vi "MultiQ_09_DataSwitch.vi"() -> ()   [LabVIEW 2021]
doc: "I. Description:\nThis example demonstrates how to acquire a finite amount of data (waveform) using the DAQ device's internal clock.\n\nII. Instructions for Running:\n1. Select the physical channel to correspond to where your signal is input on the DAQ device.\n2. Enter the minimum and maximum voltages.\nNote: For better accuracy try to match the input range to the expected voltage level of the measured signal.\n3. Select the number of samples to acquire.\n4. Set the rate of the acquisition\nNote: The rate should be AT LEAST twice as fast as the maximum frequency component of the signal being acquired.\n\nIII. Block Diagram Steps:\n Steps: \n1. Create an empty task.\n2. Create an analog input voltage channel. Use the DAQmx Base configuration Utility (Tools Menu) to determine the DAQ device name. \n3. Set the rate for the sample clock. Additionally, define the sample mode to be finite and set the number of samples to be acquired per channel.\n4. Call the Start VI to start the acquisition.\n5. Use the Read VI to measure multiple samples from N Channels on the device. Set a timeout so an error is returned if the samples are not returned in the specified time limit\n6. Stop the Analog Input Task.\n7. Call the Clear Task VI to clear the Task.\n8. Use the popup dialog box to display an error if any.\n \nIV. I/O Connections Overview:\nMake sure your signal input terminal matches the Physical Channel I/O Control. For further connection information, refer to your hardware reference manual."
uses:
  <vilib>/Utility/error.llb/DialogType.ctl
  <vilib>/DAQmx/write.llb/DAQmx Write (Analog 2D DBL NChan NSamp).vi
  <vilib>/measure/maspectr.llb/FFT Power Spectrum and PSD for 1 Chan.vi
  <vilib>/DAQmx/configure/timing.llb/DAQmx Timing (Sample Clock).vi
  <vilib>/DAQmx/miscellaneous.llb/DAQmx Fill In Error Info.vi
  <vilib>/Analysis/2dsp.llb/Decimate (continuous, DBL).vi
  <vilib>/DAQmx/create/channels.llb/DAQmx Create Channel (AI-Voltage-Basic).vi
  <vilib>/measure/macond.llb/IIR Filter for 1 Chan.vi
  <vilib>/DAQmx/configure/trigger.llb/DAQmx Start Trigger (Digital Edge).vi
  <vilib>/DAQmx/create/channels.llb/DAQmx Create Channel (AO-Voltage-Basic).vi
  <vilib>/DAQmx/read.llb/DAQmx Read (Analog 2D DBL NChan NSamp).vi
  <vilib>/measure/NI_MAPro.lvlib
  <vilib>/measure/NI_MABase.lvlib
  <vilib>/Analysis/NI_AALPro.lvlib
  <resource>/objmgr/daqmx.rc
panel:
  out "Nodal Modes":dbl[](array[numeric])=[1092.3, 1649.9, 2505.8]
  out "PlotLabelSize":i32[](array[numeric])
  out "PlotModeSize":i32[](array[numeric])
  out "PlotFreqArray":dbl[][](array[numeric])
  out "PlotLabelArray":string[][](array[string])
  out "Shear Modes":dbl[](array[numeric])=[1092.3, 1649.9, 2505.8]
  out "All Modes":dbl[](array[numeric])=[1092.3, 1649.9, 2505.8]
  out "Modes 10-12":dbl[](array[numeric])=[10072.0, 11259.0, 12454.0]
  out "Modes 7-9":dbl[](array[numeric])=[6683.3, 7225.3, 9346.1]
  in  "Sample Modes":u16(ring)=1 items=["All Modes", "Shear Modes"]
  out "Plot7Label":string="Mode 15: 15961 Hz"
  out "Plot5Label":string="Mode 9: 9346 Hz"
  out "Plot3Label":string="Mode 5: 4361 Hz"
  out "Plot1Label":string="Mode 1: 1092 Hz"
  out "Plot8Label":string="Mode 18: 19859 Hz"
  out "Plot6Label":string="Mode 12: 12454 Hz"
  out "Plot4Label":string="Mode 6: 6645 Hz"
  out "Plot2Label":string="Mode 3: 2506 Hz"
  in  "Ring":u16(ring) items=["EXCITE", "ACQUIRE", "X-Y"]
  in  "Max Value":dbl=10.0 format="%#_13g"
  in  "Min Value":dbl=-10.0 format="%#_13g"
  out "Modes 4-6":dbl[](array[numeric])=[3847.7, 4361.2, 6645.1]
  out "Modes 1-3":dbl[](array[numeric])=[1092.3, 1649.9, 2505.8]
  out "Converted Data Size":i32[](array[numeric])
  out "Raw Data Size":i32[](array[numeric])
  in  "Input Data Type":u16(ring) items=["X Y SUM", "Q 1+/- -- 4+/-", "Q 1-4"]
  in  "Mode Scale":dbl=1.0 min=0.5 max=2.0
  in  "Range (%)":dbl=1.0
  in  "Pressure (t)":sgl=1e-06
  in  "LeverArm (m)":dbl=1.0 min=1.0 max=10000.0
  in  "ADC Range":u16(ring)=6 items=["±0.1 V", "±0.2 V", "±0.5 V", "±1 V", "±2 V", "±5 V", "±10 V"]
  out "PlotLimit":u64
  out "Plot":i32
  in  "Type":u16(ring)=1 items=["Power Spectrum", "PS Density"]
  in  "Unit":u16(ring)=3 items=["Volts", "mRad (full)", "mRad (o2)", "mRad (o1)"]
  in  "Averaging":T1={"Averaging"=enum."No averaging", "weighting mode"=enum."Linear", "number of averages"=10} {"number of averages" min=1 step=1}
  out "Progress":u8(slide) scale=0.0..100.0
  in  "Who":string(combo)="SP"
  in  "fMinPlot":dbl=0.5
  in  "fMaxPlot":dbl=15.0 min=1.0 max=100.0
  in  "Substrate":u16(ring)=1 items=["Silica: 75 x 0.3 mm", "Silica: 75 x 1.0 mm", "Silica: 75 x 2.54 mm"]
  in  "Oversample":bool=TRUE
  in  "fOversample":dbl=50.0 format="%#_13g"
  in  "Span":u32(ring)=60 items=["20 s"=20, "40 s"=40, "1 min"=60, "3 min"=180, "5 min"=300]
  in  "Offset (V)":sgl=2.0
  in  "Ampl. (V)":sgl=2.0
  out "NAve":dbl format="%#_13g"
  out "ADCScale":dbl format="%#_13g"
  out "SizeTimeSeries":i32
  out "BufferPeriod":dbl format="%#_13g"
  out "PSD X":cluster{"f0":dbl, "df":dbl, dbl[][]}(graph)
  out "PlotUnitIndex":u16
  out "DataFilePath":path
  out "fSampleAcquire":dbl format="%#_13g"
  out "NDataPointsOutput":u64
  out "DeltaTOutput":dbl format="%#_13g"
  out "fSampleOutput":dbl format="%#_13g"
  out "DecimFactor":u32
  in  "Comment":string
  out "WriteNumber":i32
  out "WriteLimit":i32
  out "Step":i32
  out "Location":string
  out "PathAtOpen":path
  out "PathAtClose":path
  out "RunLight":bool
  in  "Temp Path":path
  in  "stop":bool
  out "Plot8":cluster{"f0":dbl, "df":dbl, dbl[][]}(graph)
  out "Plot7":cluster{"f0":dbl, "df":dbl, dbl[][]}(graph)
  out "WriteNewHeader":bool
  out "TempFilePath":path
  out "RunPeriod":dbl format="%#_13g"
  out "NDataPointsAcquire":u64
  out "nPlotPerRun":u64
  out "InitialArray":dbl[][](array[numeric])
  out "time vector":dbl[](array[numeric])
  out "ReZero":dbl[][](array[numeric])
  out "df":dbl format="%#_13g"
  out "PlotPeriod":dbl format="%#_13g"
  in  "Run Duration (s)":u32=100 caption="Duration (s)"
  in  "Run Number":i8=1
  in  "∆f (Hz)":u32(ring)=1 items=["1.00"=1, "0.50"=2, "0.25"=4, "0.10"=10]
  in  "Excite":bool
  out "# Elements Response Queue":i32
  out "BufferPeriod ms":u32
  out "# Elements Drive Queue":i32
  out "High Pass IIR filter specs":T2={"Topology"=enum."Butterworth", "Type"=enum."Bandpass", "Order"=7, "Lower Fc"=2000.0, "Upper Fc"=3800.0, "PB Ripple"=0.025, "SB Attenuation"=90.0}
  out "DeltaTAcquire":dbl format="%#_13g"
  out "BufferPoints":u32
  out "PlotPoints":u32
  out "nBufferPerPlot":u32
  out "fMaxPlotHz":dbl format="%#_13g"
  out "fMinPlotHz":dbl format="%#_13g"
  out "Plot6":cluster{"f0":dbl, "df":dbl, dbl[][]}(graph)
  out "Plot5":cluster{"f0":dbl, "df":dbl, dbl[][]}(graph)
  out "Plot4":cluster{"f0":dbl, "df":dbl, dbl[][]}(graph)
  out "Plot3":cluster{"f0":dbl, "df":dbl, dbl[][]}(graph)
  out "Plot2":cluster{"f0":dbl, "df":dbl, dbl[][]}(graph)
  out "Plot1":cluster{"f0":dbl, "df":dbl, dbl[][]}(graph)
  in  "Start":bool
  out "PSD Y":cluster{"f0":dbl, "df":dbl, dbl[][]}(graph) caption="Measurement"
  out "File":string
  in  "Path":path caption="File Name"
  in  "Label":string
  in  "Name":string
  out "HTML \nTitle":string
  out "Start Time":timestamp
  out "Write Light":bool
  in  "AutoSave":bool=TRUE
  in  "Manual Save":bool=TRUE caption="Saving Data"
  out "Out":path caption="File Name Out"
  in  "QUIT":bool
  # "Acquire"
  # "Multi Q\nVer 0.9.5.0 • July 2021\nSteve Penn"
  # "Sample"
  # "Comment"
  # "Frequency"
  # "kHz"
  # ":"
  # "Oversample"
  # "kHz"
  # "PLOT:"
  # "Mode Plots:"
  # "PSD Y / Excitation"
  # "/"
  # "Averaging"
  # "Drive"
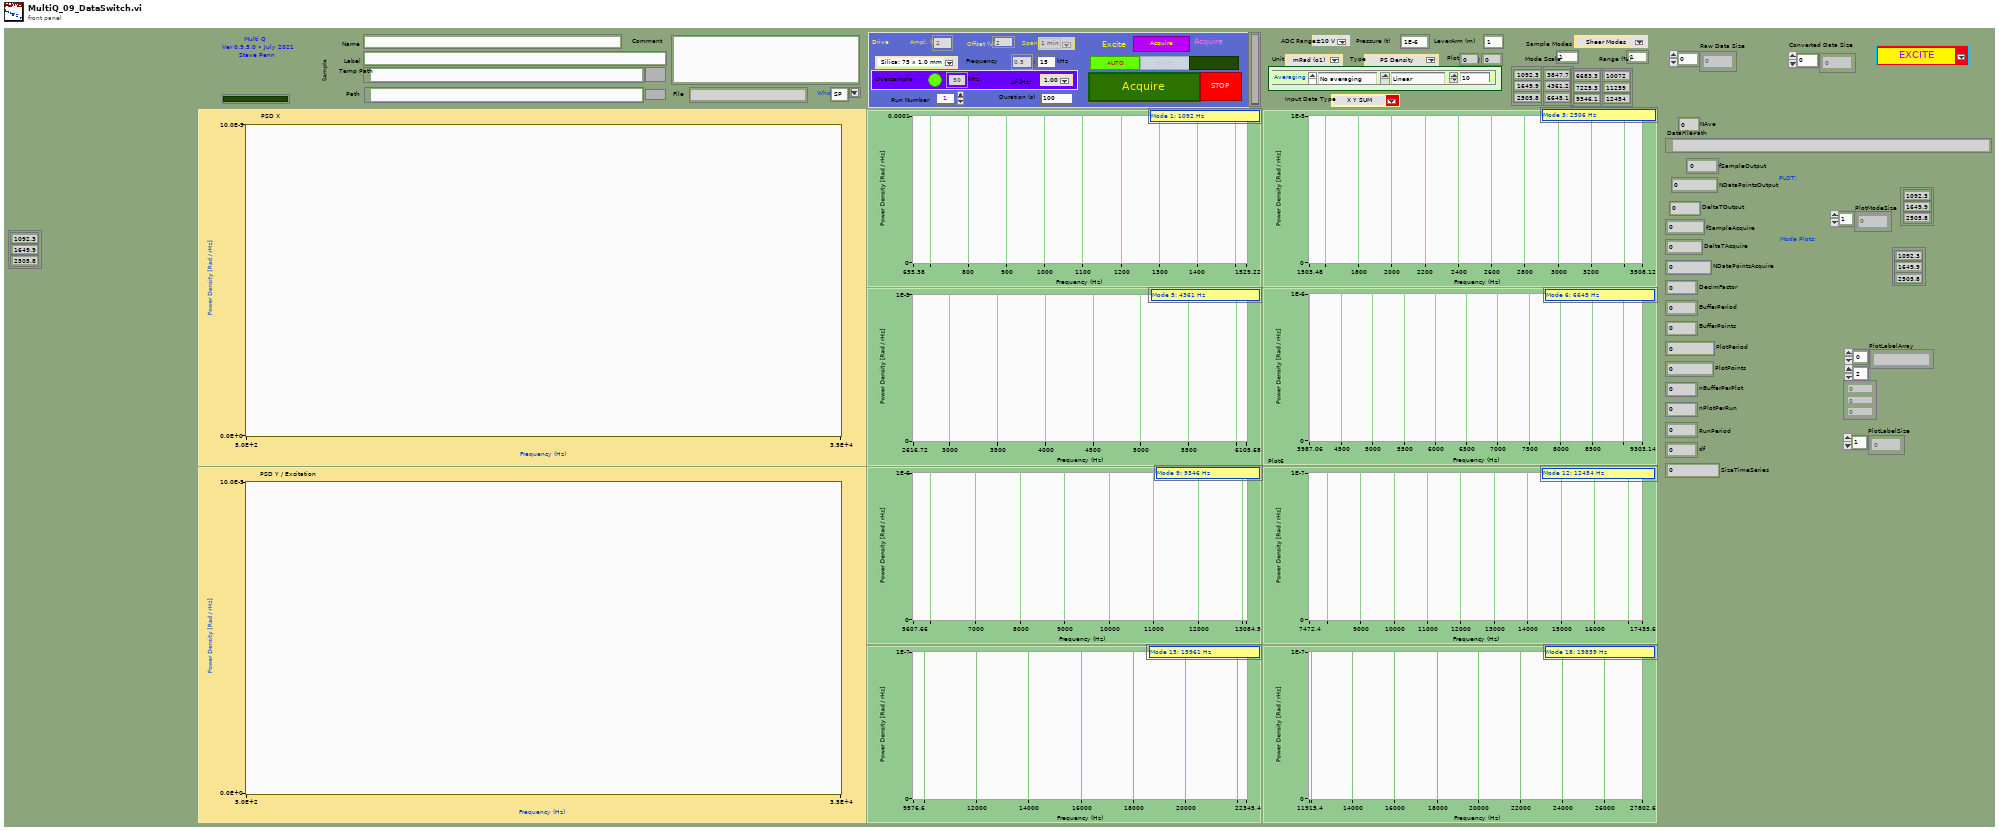
[diagram p1: front panel]
types:
  T1 = cluster{"Averaging":enum16{"No averaging", "Vector averaging", "RMS averaging", "Peak hold"}, "weighting mode":enum16{"Linear", "Exponential"}, "number of averages":u32}
  T2 = cluster{"Topology":enum16{"Off", "Butterworth", "Chebyshev", "Inverse Chebyshev", "Elliptic", "Bessel"}, "Type":enum16{"Lowpass", "Highpass", "Bandpass", "Bandstop"}, "Order":i32, "Lower Fc":dbl, "Upper Fc":dbl, "PB Ripple":dbl, "SB Attenuation":dbl}
  T3 = enum16{"Off", "Butterworth", "Chebyshev", "Inverse Chebyshev", "Elliptic", "Bessel"}
  T4 = enum16{"Lowpass", "Highpass", "Bandpass", "Bandstop"}
  T5 = enum8{"open", "replace", "create", "open or create", "replace or create", "replace or create with confirmation"}
  T6 = enum16{"No averaging", "Vector averaging", "RMS averaging", "Peak hold"}
  T7 = cluster{"Averaging":enum16{"No averaging", "Vector averaging", "RMS averaging", "Peak hold"}, "weighting mode":enum16{"Linear", "Exponential"}, "weighting mode":u64}
  T8 = typedef "DialogType.ctl" = u16
  T9 = enum16{"Left Button", "Center Button", "Right Button", "Window Close"}
  T10 = cluster{"Averaging":enum16{"No averaging", "Vector averaging", "RMS averaging", "Peak hold"}, "weighting mode":enum16{"Linear", "Exponential"}, "Value":u64}
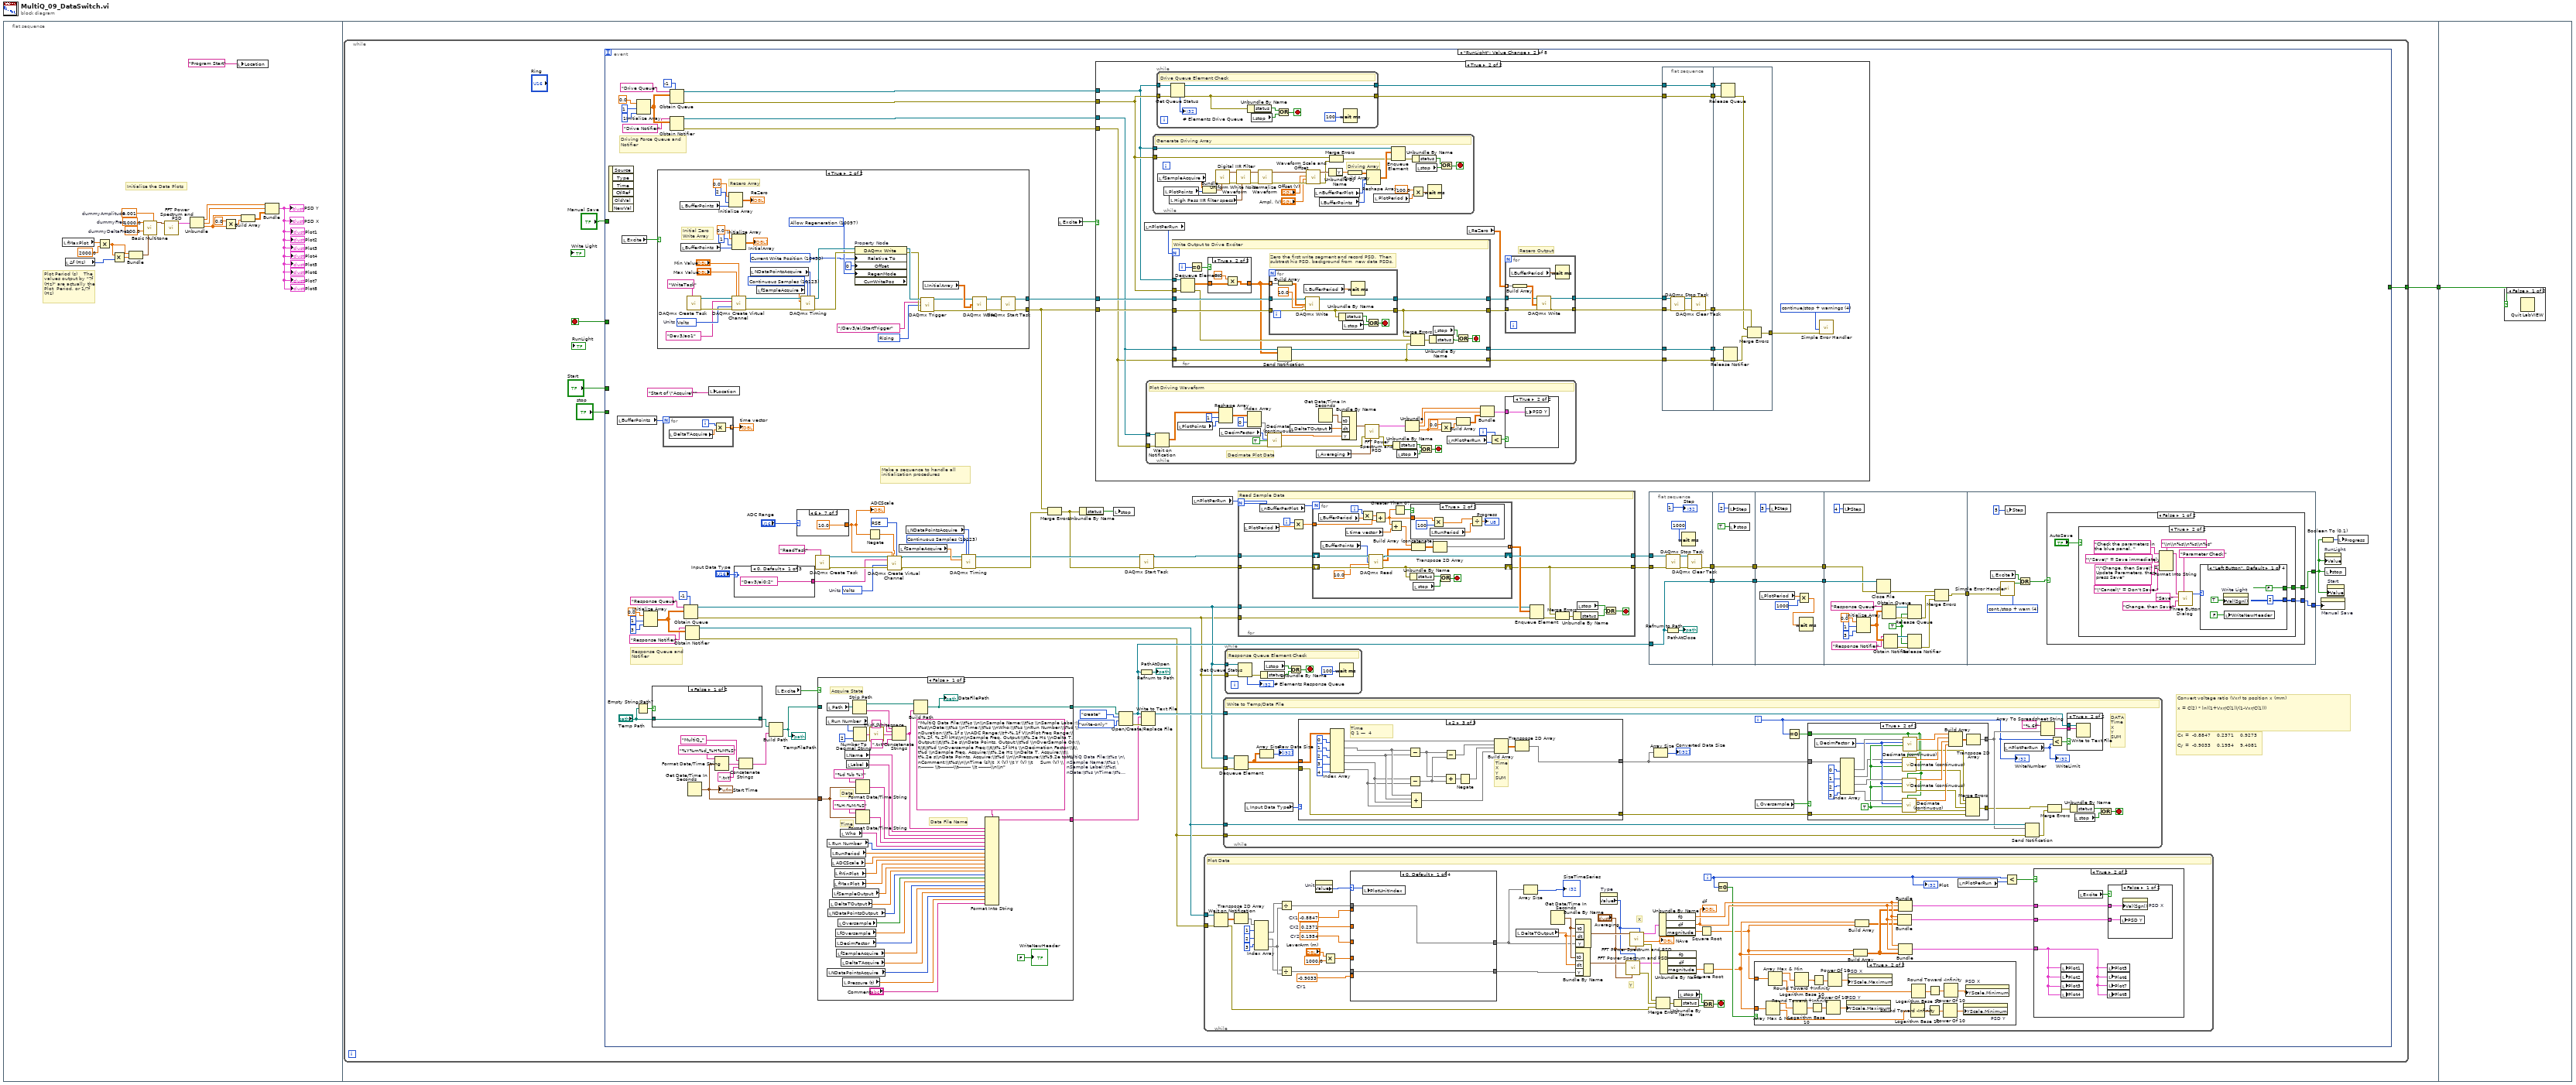
[diagram p0: block diagram]
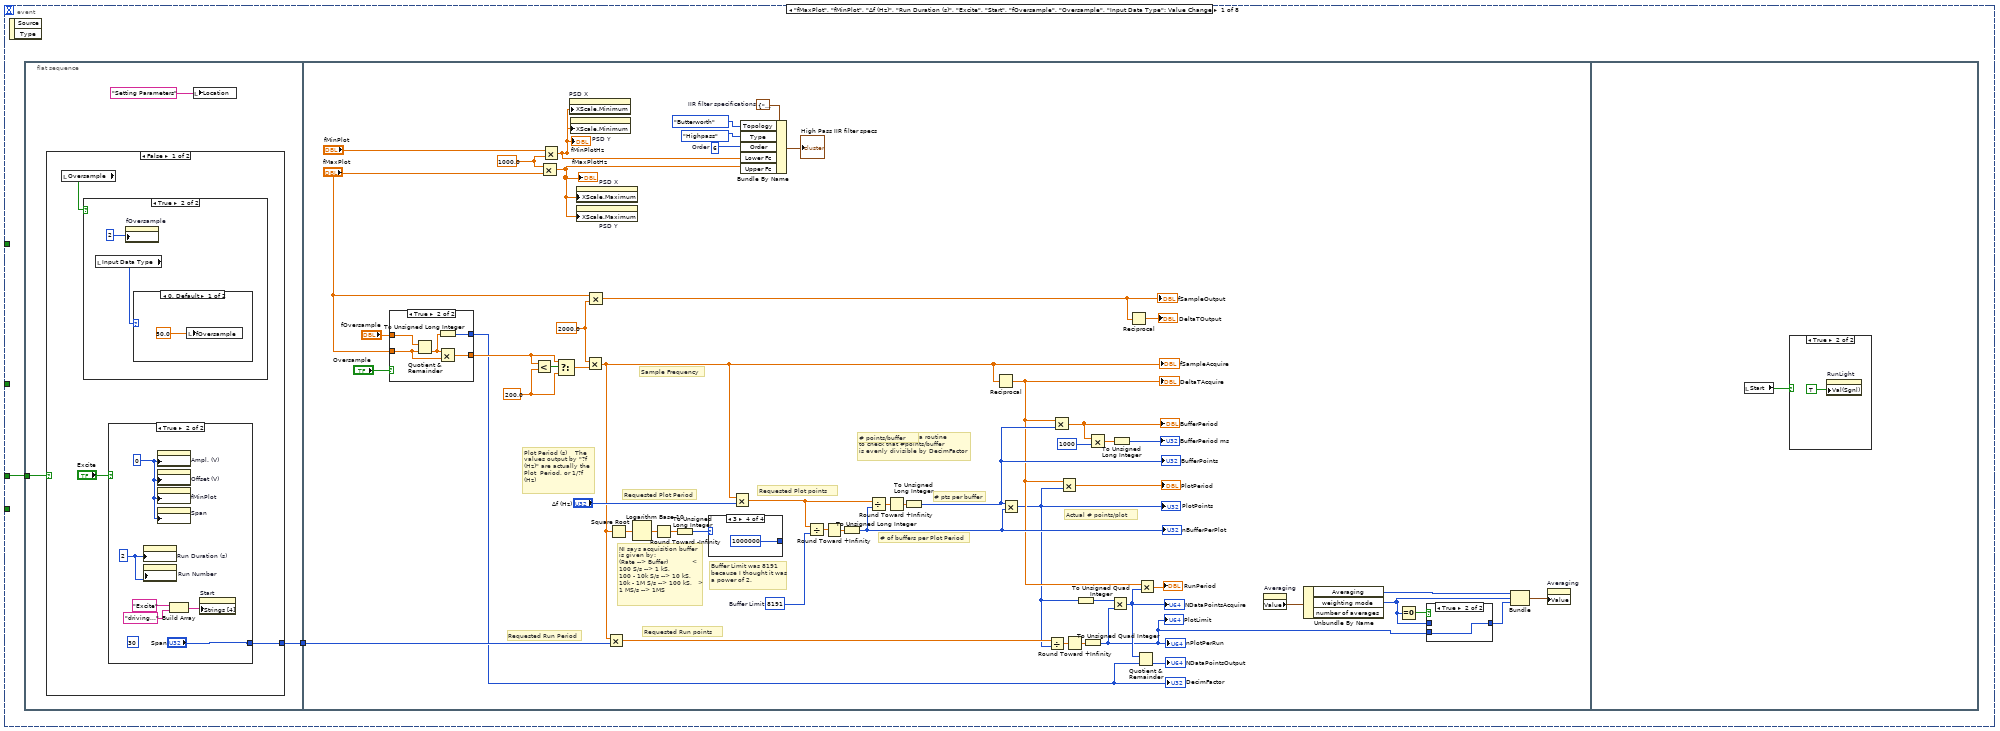
[diagram p2: hidden frame]
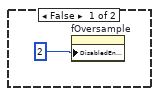
[diagram p3: hidden frame]
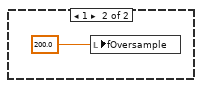
[diagram p4: hidden frame]
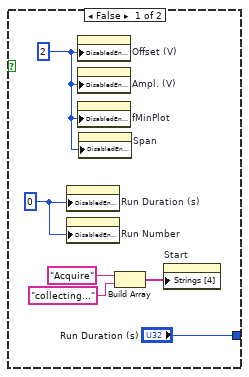
[diagram p5: hidden frame]
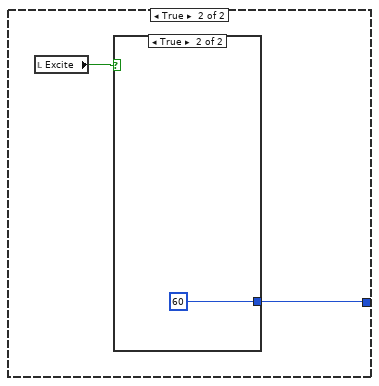
[diagram p6: hidden frame]
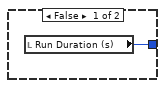
[diagram p7: hidden frame]
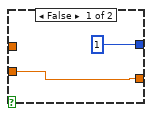
[diagram p9: hidden frame]
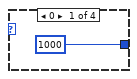
[diagram p10: hidden frame]
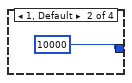
[diagram p11: hidden frame]
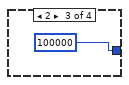
[diagram p12: hidden frame]
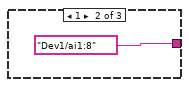
[diagram p14: hidden frame]
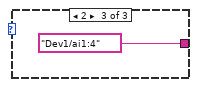
[diagram p15: hidden frame]
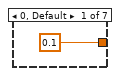
[diagram p16: hidden frame]
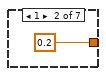
[diagram p17: hidden frame]
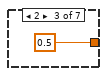
[diagram p18: hidden frame]
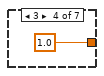
[diagram p19: hidden frame]
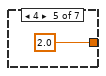
[diagram p20: hidden frame]
diagram:
  n1 = flat-sequence {
    tunnel: [w21] -> w1
    tunnel: w1 -> [w1121]
    frame #0 {
      w4 = 0.001  # dummyAmplitude
      w2 = 100.0  # dummyDeltaFreq
      w3 = 1000.0  # dummyFreq
      # "Initialize the Data Plots"
      # "Plot Period (s)    The values output by \"?f (Hz)\" are actually the Plot  Period, or 1/?f (Hz)"
      n2 = local read "fMaxPlot"() -> (w9:dbl)
      n3 = local read "∆f (Hz)"() -> (w8:u32)
      n4 = Multiply(x=w9, y=2000.0) -> (x*y=w6:dbl)
      n5 = Multiply(x=w6, y=w8) -> (x*y=w7:dbl)
      n6 = Bundle(w6, w7) -> (w19:cluster{dbl, dbl})  [unwired: 1 in]
      n7 = call <vilib>:"Basic Multitone.vi"("start frequency"=w3, "amplitude"=w4, "delta frequency"=w2, "sampling info"=w19) -> ("signal out"=w18:waveform(dbl))  [unwired: 8 in, 3 out]
      n8 = call-poly <vilib>:"FFT Power Spectrum and PSD.vi"("time signal"=w18) -> ("Power Spectrum / PSD"=w11:cluster{"f0":dbl, "df":dbl, "magnitude":dbl[]})  [unwired: 7 in, 3 out]
      n9 = Unbundle(w11) -> ("f0"=w16:dbl, "df"=w13:dbl, "magnitude"=w12:dbl[])
      n10 = Multiply(x=0.0, y=w12) -> (x*y=w14:dbl[])
      n11 = local write "Location"("Program Start") -> ()
      n12 = Build Array(w12, w14) -> (w15:dbl[][])
      n13 = Bundle("f0"=w16, "df"=w13, w15) -> (→"PSD Y" →"PSD X" →"Plot5" →"Plot6" →"Plot7" →"Plot8" →"Plot3" →"Plot1" →"Plot2" →"Plot4":cluster{"f0":dbl, "df":dbl, dbl[][]})  [unwired: 1 in]
    }
    frame #1 {
      n14 = while {
        tunnel: [w25] -> w21
        stop <- w26 stop-if-true
        n15 = event shown="[1] \"RunLight\": Value Change" {
          selector: _ -> [_ _ _ _ _ _ _ _]
          dyn-events: _ -> [_ _ _ _ _ _ _ _]
          timeout: _ -> [_ _ _ _ _ _ _ _]
          tunnel: [_ _ _ _ _ _ w1096 _] -> w26
          tunnel: [_ _ _ _ _ _ w1097 _] -> w25
          tunnel: "Manual Save" -> [_ _ _ _ _ _ _ _]
          tunnel: "Start" -> [w27 _ _ _ _ _ _ _]
          tunnel: "stop" -> [_ _ _ _ _ _ _ _]
          event "fMaxPlot", "fMinPlot", "∆f (Hz)", "Run Duration (s)", "Excite", "Start", "fOversample", "Oversample", "Input Data Type": Value Change {
            n16 = event-data() -> ()  [unwired: 3 out]
            n17 = flat-sequence {
              tunnel: [w31] -> w28
              tunnel: w27 -> [w30]
              tunnel: w28 -> [w77]
              frame #0 {
                n18 = case shown="False" w30 {
                  tunnel: [w33 w52] -> w31
                  frame False {
                    n19 = local read "Oversample"() -> (w32:bool)
                    n20 = case shown="True" w32 {
                      frame False {
                        n21 = property on="fOversample" class="DigNum (strict)"("DisabledEnum"=2) -> ()  [unwired: 2 in, 2 out]
                      }
                      frame True {
                        n22 = local read "Input Data Type"() -> (w36:u16)
                        n23 = property on="fOversample" class="DigNum (strict)"("DisabledEnum"=2) -> ()  [unwired: 2 in, 2 out]
                        n24 = case shown="0, Default" w36 {
                          frame 0, Default {
                            n25 = local write "fOversample"(50.0) -> ()
                          }
                          frame 1 {
                            n26 = local write "fOversample"(200.0) -> ()
                          }
                        }
                      }
                    }
                    n27 = case shown="True" "Excite" {
                      tunnel: ["Run Duration (s)" "Span"] -> w33
                      frame False {
                        w42 = 0
                        w40 = 2
                        n28 = property on="Run Duration (s)" class="DigNum (strict)"("DisabledEnum"=w42) -> ()  [unwired: 2 in, 2 out]
                        n29 = property on="Run Number" class="DigNum (strict)"("DisabledEnum"=w42) -> ()  [unwired: 2 in, 2 out]
                        n30 = property on="Offset (V)" class="DigNum (strict)"("DisabledEnum"=w40) -> ()  [unwired: 2 in, 2 out]
                        n31 = property on="Ampl. (V)" class="DigNum (strict)"("DisabledEnum"=w40) -> ()  [unwired: 2 in, 2 out]
                        n32 = property on="fMinPlot" class="DigNum (strict)"("DisabledEnum"=w40) -> ()  [unwired: 2 in, 2 out]
                        n33 = property on="Span" class="Ring (strict)"("DisabledEnum"=w40) -> ()  [unwired: 2 in, 2 out]
                        n34 = Build Array("Acquire", "collecting...") -> (w45:string[])
                        n35 = property on="Start" class="Bool (strict)"("Strings [4]"=w45) -> ()  [unwired: 2 in, 2 out]
                      }
                      frame True {
                        (unwired) 30
                        w48 = 2
                        w47 = 0
                        n36 = property on="Run Duration (s)" class="DigNum (strict)"("DisabledEnum"=w48) -> ()  [unwired: 2 in, 2 out]
                        n37 = property on="Run Number" class="DigNum (strict)"("DisabledEnum"=w48) -> ()  [unwired: 2 in, 2 out]
                        n38 = property on="Ampl. (V)" class="DigNum (strict)"("DisabledEnum"=w47) -> ()  [unwired: 2 in, 2 out]
                        n39 = property on="Offset (V)" class="DigNum (strict)"("DisabledEnum"=w47) -> ()  [unwired: 2 in, 2 out]
                        n40 = property on="fMinPlot" class="DigNum (strict)"("DisabledEnum"=w47) -> ()  [unwired: 2 in, 2 out]
                        n41 = property on="Span" class="Ring (strict)"("DisabledEnum"=w47) -> ()  [unwired: 2 in, 2 out]
                        n42 = Build Array("Excite", "driving...") -> (w51:string[])
                        n43 = property on="Start" class="Bool (strict)"("Strings [4]"=w51) -> ()  [unwired: 2 in, 2 out]
                      }
                    }
                  }
                  frame True {
                    n44 = local read "Excite"() -> (w53:bool)
                    n45 = case shown="True" w53 {
                      tunnel: [w54 60] -> w52
                      frame False {
                        n46 = local read "Run Duration (s)"() -> (w54:u32)
                      }
                      frame True {
                      }
                    }
                  }
                }
                n47 = local write "Location"("Setting Parameters") -> ()
              }
              frame #1 {
                w98 = 6  # Order
                w101 = T2 {"Topology"=enum."Butterworth", "Type"=enum."Bandpass", "Order"=7, "Lower Fc"=2000.0, "Upper Fc"=3800.0, "PB Ripple"=0.025, "SB Attenuation"=90.0}  # IIR filter specifications
                w107 = 1000.0
                w87 = 8191  # Buffer Limit
                w74 = 2000.0
                w106 = 200.0
                # "# pts per buffer"
                # "I may need to add a routine \nto check that #points/buffer\nis evenly divisible by DecimFactor"
                # "Requested Run points"
                # "Requested Run Period"
                # "Requested Plot Period"
                # "NI says acquisition buffer  is given by:                   (Rate --> Buffer)            < 100 S/s --> 1 kS,                 100 - 10k S/s --> 10 kS,   10k - 1M S/s --> 100 kS,   > 1 MS/s --> 1MS"
                # "Buffer Limit was 8191 because I thought it was a power of 2."
                # "Plot Period (s)    The values output by \"?f (Hz)\" are actually the Plot  Period, or 1/?f (Hz)"
                # "Sample Frequency"
                # "Actual # points/plot"
                # "# points/buffer"
                # "Requested Plot points"
                # "# of buffers per Plot Period"
                n48 = case shown="True" "Oversample" {
                  tunnel: "fOversample" -> [_ w120]
                  tunnel: [w115 w119] -> w75
                  tunnel: "fMaxPlot" -> [w115 w118]
                  tunnel: [1 w117] -> w67
                  frame False {
                  }
                  frame True {
                    n49 = Quotient & Remainder(x=w120, y=w118) -> (floor(x/y)=w116:dbl)  [unwired: 1 out]
                    n50 = Multiply(x=w116, y=w118) -> (x*y=w119:dbl)
                    n51 = To Unsigned Long Integer(number=w116) -> (unsigned 32bit integer=w117:u32)
                  }
                }
                "DecimFactor" <- w67
                n52 = Less?(x=w75, y=w106) -> (x < y?=w111:bool)
                n53 = Multiply(x=w107, y="fMaxPlot") -> (x*y=w65:dbl)
                "fMaxPlotHz" <- w65
                n54 = Multiply(x="fMinPlot", y=w107) -> (x*y=w66:dbl)
                "fMinPlotHz" <- w66
                n55 = Select(t=w75, s=w111, f=w106) -> (s? t:f=w110:dbl)
                n56 = property on="PSD X" class="WFGraph (strict)"("XScale.Minimum"=w66) -> ()  [unwired: 2 in, 2 out]
                n57 = property on="PSD Y" class="WFGraph (strict)"("XScale.Minimum"=w66) -> ()  [unwired: 2 in, 2 out]
                n58 = property on="PSD X" class="WFGraph (strict)"("XScale.Maximum"=w65) -> ()  [unwired: 2 in, 2 out]
                n59 = property on="PSD Y" class="WFGraph (strict)"("XScale.Maximum"=w65) -> ()  [unwired: 2 in, 2 out]
                n60 = Multiply(x=w74, y=w110) -> (x*y=w84:dbl)
                "fSampleAcquire" <- w84
                n61 = Multiply(x="fMaxPlot", y=w74) -> (x*y=w72:dbl)
                "fSampleOutput" <- w72
                n62 = Multiply(x=w84, y=w77) -> (x*y=w83:dbl)
                n63 = Square Root(x=w84) -> (sqrt(x)=w92:dbl)
                n64 = Logarithm Base 10(1:w92) -> (0:w91:dbl)
                n65 = Round Toward -Infinity(1:w91) -> (0:w90:dbl)
                n66 = To Unsigned Long Integer(number=w90) -> (unsigned 32bit integer=w89:u32)
                n67 = case shown="3" w89 {
                  tunnel: [1000 10000 100000 1000000] -> _
                  frame 0 {
                  }
                  frame 1, Default {
                  }
                  frame 2 {
                  }
                  frame 3 {
                  }
                }
                n68 = Multiply(x=w84, y="∆f (Hz)") -> (x*y=w109:dbl)
                n69 = Bundle By Name(cluster=w101, "Topology"=T3."Butterworth", "Type"=T4."Highpass" ("Enum"), "Order"=w98, "Lower Fc"=w66, "Upper Fc"=w65) -> (→"High Pass IIR filter specs":T2)
                n70 = Divide(x=w109, y=w87) -> (x/y=w105:dbl)
                n71 = Round Toward +Infinity(x=w105) -> (ceil(x): smallest int >= x=w104:dbl)
                n72 = To Unsigned Long Integer(number=w104) -> (unsigned 32bit integer=w102:u32)
                "nBufferPerPlot" <- w102
                n73 = Divide(x=w109, y=w102) -> (x/y=w108:dbl)
                n74 = Round Toward +Infinity(x=w108) -> (ceil(x): smallest int >= x=w103:dbl)
                n75 = To Unsigned Long Integer(number=w103) -> (unsigned 32bit integer=w80:u32)
                "BufferPoints" <- w80
                n76 = Reciprocal(x=w84) -> (1/x=w79:dbl)
                "DeltaTAcquire" <- w79
                n77 = Multiply(x=w80, y=w102) -> (x*y=w56:u32)
                "PlotPoints" <- w56
                n78 = Divide(x=w83, y=w56) -> (x/y=w82:dbl)
                n79 = Multiply(x=w79, y=w80) -> (x*y=w95:dbl)
                "BufferPeriod" <- w95
                n80 = Multiply(x=w79, y=w56) -> (x*y=→"PlotPeriod":dbl)
                n81 = Round Toward +Infinity(x=w82) -> (ceil(x): smallest int >= x=w81:dbl)
                n82 = To Unsigned Quad Integer(1:w56) -> (0:w57:u64)
                n83 = To Unsigned Quad Integer(1:w81) -> (0:w58:u64)
                "nPlotPerRun" <- w58
                "PlotLimit" <- w58
                n84 = Multiply(x=w95, y=1000) -> (x*y=w94:dbl)
                n85 = Multiply(x=w57, y=w58) -> (x*y=w70:u64)
                "NDataPointsAcquire" <- w70
                n86 = To Unsigned Long Integer(number=w94) -> (unsigned 32bit integer=→"BufferPeriod ms":u32)
                n87 = Reciprocal(x=w72) -> (1/x=→"DeltaTOutput":dbl)
                n88 = Quotient & Remainder(x=w70, y=w67) -> (floor(x/y)=→"NDataPointsOutput":u64)  [unwired: 1 out]
                n89 = Multiply(x=w79, y=w70) -> (x*y=→"RunPeriod":dbl)
                n90 = property on="Averaging" class="Clust (strict)"() -> ("Value"=w60:T1)  [unwired: 2 in, 2 out]
                n91 = Unbundle By Name(w60) -> ("Averaging"=w61:T6, "weighting mode"=w64:enum16{"Linear", "Exponential"})  [unwired: 1 out]
                n92 = Equal To 0?(x=w64) -> (x = 0?=w62:bool)
                n93 = case shown="True" w62 {
                  tunnel: [w112 w113] -> w63
                  tunnel: w64 -> [w112 _]
                  tunnel: w58 -> [_ w113]
                  frame False {
                  }
                  frame True {
                  }
                }
                n94 = Bundle("Averaging"=w61, "weighting mode"=w64, "weighting mode"=w63) -> (w59:T7)  [unwired: 1 in]
                n95 = property on="Averaging" class="Clust (strict)"("Value"=w59) -> ()  [unwired: 2 in, 2 out]
              }
              frame #2 {
                n96 = local read "Start"() -> (w125:bool)
                n97 = case shown="True" w125 {
                  frame False {
                  }
                  frame True {
                    n98 = property on="RunLight" class="Bool (strict)"("Val(Sgnl)"=TRUE) -> ()  [unwired: 2 in, 2 out]
                  }
                }
              }
            }
          }
          event "RunLight": Value Change {
            w135 = 10123 items=["Finite Samples"=10178, "Continuous Samples"=10123] ("sample mode")
            w138 = 10348 items=["Volts"=10348]  # Units
            w143 = 10083 items=["default"=-1, "differential"=10106, "RSE"=10083, "NRSE"=10078] ("input terminal configuration")
            # "Cx =  -0.8847    0.2371    0.9273\n\nCy =  -0.9033    0.1954    9.4081"
            # "Convert voltage ratio (Vxr) to position x (mm)\n\nx = C(2) * ln((1+Vxr/C(1))/(1-Vxr/C(1)))"
            # "Response Queue and Notifier"
            # "Driving Force Queue and Notifier"
            # "Make a sequence to handle all initialization procedures"
            n99 = event-data() -> ()  [unwired: 7 out]
            n100 = local read "BufferPoints"() -> (w199:u32)
            n101 = local read "Excite"() -> (w196:bool)
            n102 = Empty String/Path?(string/path="Temp Path") -> (empty?=w184:bool)
            n103 = Initialize Array(0.0, 1, 1) -> (w173:dbl[][])
            n104 = Initialize Array(0.0, 1, 3) -> (w162:dbl[][])
            n105 = case shown="False" w184 {
              tunnel: "Temp Path" -> [w477 _]
              tunnel: [w477 w478] -> w182
              frame False {
              }
              frame True {
                w478 = path "/Users/qlab/Documents/MultiQ/Temp"
                n106 = local write "Temp Path"(w478) -> ()
              }
            }
            n107 = case shown="True" w196 {
              tunnel: [w684 w691] -> w195
              tunnel: [w685 w692] -> w197
              frame False {
                n108 = call <vilib>:"DAQmx Create Task.vi"() -> ("task out"=w685:refnum<k21>, "error out"=w684:errorcluster)  [unwired: 14 in]
              }
              frame True {
                w687 = 10430 items=["First Sample"=10424, "Current Write Position"=10430] ("RelativeTo")
                w700 = 10097 items=["Allow Regeneration"=10097, "Do Not Allow Regeneration"=10158] ("RegenMode")
                w696 = 10280 items=["Falling"=10171, "Rising"=10280]
                w704 = 10123 items=["Finite Samples"=10178, "Continuous Samples"=10123] ("sample mode")
                w708 = 10348 items=["Volts"=10348]  # Units
                # "Initial Zero Write Array"
                # "Rezero Array"
                n109 = local read "BufferPoints"() -> (w719:u32)
                n110 = local read "BufferPoints"() -> (w717:u32)
                n111 = call <vilib>:"DAQmx Create Task.vi"("new task name"="WriteTask") -> ("task out"=w710:refnum<k21>, "error out"=w709:errorcluster)  [unwired: 13 in]
                n112 = Initialize Array(0.0, 2, w719) -> (→"ReZero":dbl[][])
                n113 = Initialize Array(0.0, 1, w717) -> (→"InitialArray":dbl[][])
                n114 = call-poly <vilib>:"DAQmx Create Virtual Channel.vi"("task in"=w710, "maximum value"="Max Value", "minimum value"="Min Value", "physical channels"=tag "Dev3/ao1", "units"=w708, "error in"=w709) -> ("task out"=w707:refnum<k21>, "error out"=w706:errorcluster)  [unwired: 8 in]
                n115 = local read "NDataPointsAcquire"() -> (w703:u64)
                n116 = local read "fSampleAcquire"() -> (w705:dbl)
                n117 = call-poly <vilib>:"DAQmx Timing.vi"("task/channels in"=w707, "sample mode"=w704, "samples per channel"=w703, "rate"=w705, "error in"=w706) -> ("task out"=w702:refnum<k21>, "error out"=w701:errorcluster)  [unwired: 9 in]
                n118 = property on="Property Node" class="DAQmx Write" props=["Relative To", "Offset", "RegenMode", "CurrWritePos"](reference=w702, error in=w701, "Relative To"=w687, "Offset"=0, "RegenMode"=w700) -> (reference out=w699:refnum<k21>, error out=w698:errorcluster)  [unwired: 1 out]
                n119 = call-poly <vilib>:"DAQmx Trigger.vi"("task/channels in"=w699, "source"=tag "/Dev3/ai/StartTrigger" ("DAQmx Terminal"), "edge"=w696, "error in"=w698) -> ("task out"=w694:refnum<k21>, "error out"=w693:errorcluster)  [unwired: 10 in]
                n120 = local read "InitialArray"() -> (w695:dbl[][])
                n121 = call-poly <vilib>:"DAQmx Write.vi"("task/channels in"=w694, "data"=w695, "error in"=w693) -> ("task out"=w689:refnum<k21>, "error out"=w690:errorcluster)  [unwired: 10 in, 1 out]
                n122 = call <vilib>:"DAQmx Start Task.vi"("task/channels in"=w689, "error in"=w690) -> ("task out"=w692:refnum<k21>, "error out"=w691:errorcluster)  [unwired: 12 in]
              }
            }
            n123 = for {
              N: w199 -> [_]
              tunnel: [w809] -> w198 mode=indexing
              i -> [w807]
              n124 = local read "DeltaTAcquire"() -> (w808:dbl)
              n125 = Multiply(x=w807, y=w808) -> (x*y=w809:dbl)
            }
            "time vector" <- w198
            n126 = Obtain Queue(max queue size (-1, unlimited)=-1, name (unnamed)="Drive Queue", element data type=w173) -> (queue out=w164:refnum<queue>, error out=w163:errorcluster)  [unwired: 2 in, 1 out]
            n127 = Obtain Notifier(name (unnamed)="Drive Notifier", notification data type=w173) -> (notifier out=w166:refnum<notifier>, error out=w165:errorcluster)  [unwired: 2 in, 1 out]
            n128 = Obtain Queue(max queue size (-1, unlimited)=-1, name (unnamed)="Response Queue", element data type=w162) -> (queue out=w154:refnum<queue>, error out=w153:errorcluster)  [unwired: 2 in, 1 out]
            n129 = Obtain Notifier(name (unnamed)="Response Notifier", notification data type=w162) -> (notifier out=w152:refnum<notifier>, error out=w151:errorcluster)  [unwired: 2 in, 1 out]
            n130 = Get Date/Time In Seconds() -> (seconds since 1Jan1904=w181:timestamp)
            "Start Time" <- w181
            n131 = local write "Location"("Start of \"Acquire\"") -> ()
            n132 = Format Date/Time String(time format string (%c)="%Y%m%d_%H%M%S", seconds (now)=w181) -> (date/time string=w207:string)  [unwired: 1 in]
            n133 = case shown="0, Default" "Input Data Type" {
              tunnel: [tag "Dev3/ai0:2" ("DAQmx Physical Channel") tag "Dev1/ai1:8" ("DAQmx Physical Channel") tag "Dev1/ai1:4" ("DAQmx Physical Channel")] -> w137
              frame 0, Default {
              }
              frame 1 {
              }
              frame 2 {
              }
            }
            n134 = Concatenate Strings("MultiQ_", w207, ".txt") -> (w186:string)
            n135 = Build Path(base path=w182, name or relative path=w186) -> (appended path=w185:path)
            "TempFilePath" <- w185
            n136 = local read "Excite"() -> (w193:bool)
            n137 = case shown="6" "ADC Range" {
              tunnel: [0.1 ("Max Value") 0.2 ("Max Value") 0.5 ("Max Value") 1.0 ("Max Value") 2.0 ("Max Value") 5.0 ("Max Value") 10.0 ("Max Value")] -> w142
              frame 0, Default {
              }
              frame 1 {
              }
              frame 2 {
              }
              frame 3 {
              }
              frame 4 {
              }
              frame 5 {
              }
              frame 6 {
              }
            }
            "ADCScale" <- w142
            n138 = call <vilib>:"DAQmx Create Task.vi"("new task name"="ReadTask") -> ("task out"=w140:refnum<k21>, "error out"=w139:errorcluster)  [unwired: 13 in]
            n139 = case shown="False" w193 {
              tunnel: [w496 w520] -> w202
              tunnel: w181 -> [w505 w519]
              tunnel: [w495 w518] -> w192
              tunnel: w185 -> [_ w518]
              frame False {
                w504 = "MultiQ Data File:\\t%s \\n\\nSample Name:\\t%s \\nSample Label:\\t%s\\nDate:\\t%s \\nTime:\\t%s \\nWho:\\t%s \\nRun Number:\\t%d \\nDuration:\\t%.1f s \\nADC Range:\\t+-%.1f V\\nPlot Freq Range:\\t(%.2f, %.2f) kHz\\n\\nSample Freq, Output:\\t%.2e Hz \\nDelta T, Output:\\t\\t%.2e s\\nData Points, Output:\\t%d \\nOverSample On:\\t\\t\\t%d \\nOversample Freq:\\t\\t%.1f kHz \\nDecimation Factor:\\t\\t%d \\nSample Freq, Acquire:\\t%.2e Hz \\nDelta T, Acquire:\\t\\t%.2e s\\nData Points, Acquire:\\t%d \\n\\nPressure:\\t%9.2e torr\\nComment:\\t%s\\n\\nTime (s)\\t  X (V) \\t Y (V) \\t     Sum (V) \\n-------- \\t---------\\t-------- \\t --------\\n\\n"  # MultiQ Data File:\t%s \n\nSample Name:\t%s \nSample Label:\t%s\nDate:\t%s \nTime:\t%s \nWho:\t%s \nRun Number:\t%d \nDuration:\t%.1f s \nADC Range:\t+-%.1f V\nPlot Freq Range:\t(%.2f, %.2f) kHz\n\nSample Freq, Output:\t%.2e Hz \nDelta T, Output:\t\t%.2e s\nData Points, Output:\t%d \nOverSample On:\t\t\t%d \nOversample Freq:\t\t%.1f kHz \nDecimation Factor:\t\t%d \nSample Freq, Acquire:\t%.2e Hz \nDelta T, Acquire:\t\t%.2e s\nData Points, Acquire:\t%d \n\nPressure:\t%9.2e torr\nComment:\t%s\n\nTime (s)\t  X (V) \t Y (V) \t     Sum (V) \n-------- \t---------\t-------- \t --------\n\n
                # "Data File Name"
                # "Date"
                # "Time"
                # "Acquire State"
                n140 = local read "Run Number"() -> (w509:i8)
                n141 = local read "NDataPointsAcquire"() -> (w481:u64)
                n142 = local read "Path"() -> (w508:path)
                n143 = local read "Run Number"() -> (w503:i8)
                n144 = local read "NDataPointsOutput"() -> (w488:u64)
                n145 = local read "DeltaTOutput"() -> (w487:dbl)
                n146 = local read "RunPeriod"() -> (w497:dbl)
                n147 = local read "ADCScale"() -> (w492:dbl)
                n148 = local read "fSampleOutput"() -> (w489:dbl)
                n149 = local read "fMaxPlot"() -> (w490:dbl)
                n150 = local read "fMinPlot"() -> (w491:dbl)
                n151 = local read "fOversample"() -> (w485:dbl)
                n152 = local read "DecimFactor"() -> (w484:u32)
                n153 = local read "fSampleAcquire"() -> (w483:dbl)
                n154 = local read "Oversample"() -> (w486:bool)
                n155 = local read "Who"() -> (w493:string)
                n156 = local read "DeltaTAcquire"() -> (w482:dbl)
                n157 = local read "Pressure (t)"() -> (w480:sgl)
                n158 = local read "Name"() -> (w499:string)
                n159 = local read "Label"() -> (w500:string)
                n160 = Strip Path(path=w508) -> (stripped path=w514:path, name=w511:string)
                n161 = Number To Decimal String(number=w509, width (-)=2) -> (decimal integer string=w515:string)
                n162 = Format Date/Time String(time format string (%c)="%d %b %Y", seconds (now)=w505) -> (date/time string=w501:string)  [unwired: 1 out]
                n163 = Format Date/Time String(time format string (%c)="%H:%M:%S", seconds (now)=w505) -> (date/time string=w502:string)  [unwired: 1 out]
                n164 = call <vilib>:"Trim Whitespace.vi"("string"=w515) -> ("trimmed string"=w512:string)  [unwired: 1 in]
                n165 = Concatenate Strings(w511, "_", w512, ".txt") -> (w498:string)
                n166 = Build Path(base path=w514, name or relative path=w498) -> (appended path=w495:path)
                "DataFilePath" <- w495
                n167 = Format Into String(format string=w504, w498, w499, w500, w501, w502, w493, w503, w497, w492, w491, w490, w489, w487, w488, w486, w485, w484, w483, w482, w481, w480, "Comment") -> (resulting string=w496:string)  [unwired: 2 in, 1 out]
                "WriteNewHeader" <- FALSE
              }
              frame True {
                # "Exciter State"
                # "Date"
                # "Time"
                n168 = Format Date/Time String(time format string (%c)="%d %b %Y", seconds (now)=w519) -> (date/time string=w522:string)  [unwired: 1 out]
                n169 = Format Date/Time String(time format string (%c)="%H:%M:%S", seconds (now)=w519) -> (date/time string=w521:string)  [unwired: 1 out]
                n170 = local write "WriteNewHeader"(FALSE) -> ()
                n171 = Format Into String(format string="Date:\\t%s \\nTime:\\t %s \\n\\nTime (s)\\t  X (V) \\t Y (V) \\t     Sum (V) \\n-------- \\t---------\\t-------- \\t --------\\n\\n", w522, w521) -> (resulting string=w520:string)  [unwired: 2 in, 1 out]
              }
            }
            n172 = Negate(x=w142) -> (-x=w141:dbl)
            n173 = call-poly <vilib>:"DAQmx Create Virtual Channel.vi"("task in"=w140, "maximum value"=w142, "minimum value"=w141, "input terminal configuration"=w143, "physical channels"=w137, "units"=w138, "error in"=w139) -> ("task out"=w133:refnum<k21>, "error out"=w132:errorcluster)  [unwired: 7 in]
            n174 = local read "fSampleAcquire"() -> (w134:dbl)
            n175 = local read "NDataPointsAcquire"() -> (w136:u64)
            n176 = call-poly <vilib>:"DAQmx Timing.vi"("task/channels in"=w133, "sample mode"=w135, "samples per channel"=w136, "rate"=w134, "error in"=w132) -> ("task out"=w130:refnum<k21>, "error out"=w131:errorcluster)  [unwired: 9 in]
            n177 = Merge Errors(w195, w131) -> (w129:errorcluster)
            n178 = local read "Excite"() -> (w194:bool)
            n179 = Unbundle By Name(w129) -> ("status"=w187:bool)
            n180 = case shown="True" w194 {
              tunnel: w197 -> [w527 w548]
              tunnel: w195 -> [w526 w547]
              tunnel: w163 -> [w530 w546]
              tunnel: w166 -> [w529 w545]
              tunnel: w165 -> [w528 w544]
              tunnel: w164 -> [w531 w542]
              frame False {
                n181 = Release Queue(queue=w531, error in (no error)=w530) -> ()  [unwired: 1 in, 3 out]
                n182 = Release Notifier(notifier=w529, error in (no error)=w528) -> ()  [unwired: 1 in, 3 out]
                n183 = call <vilib>:"DAQmx Clear Task.vi"("task in"=w527, "error in"=w526) -> ()  [unwired: 13 in, 1 out]
              }
              frame True {
                w543 = T8 4 items=["no dialog", "OK message", "continue or stop message", "OK message + warnings", "continue/stop + warnings"] ("type of dialog (OK msg:1)")
                # "Rezero Output"
                n184 = local read "nPlotPerRun"() -> (w554:u64)
                n185 = while {
                  tunnel: w545 -> [w603]
                  tunnel: w544 -> [w602]
                  i -> [w589]
                  stop <- w591 stop-if-true
                  # "Decimate Plot Data"
                  # "Plot Driving Waveform"
                  n186 = Wait on Notification(notifier=w603, error in (no error)=w602) -> (notification=w601:dbl[][], error out=w580:errorcluster)  [unwired: 2 in, 2 out]
                  n187 = local read "PlotPoints"() -> (w599:u32)
                  n188 = Reshape Array(w601, 1, w599) -> (w598:dbl[][])
                  n189 = local read "DecimFactor"() -> (w586:u32)
                  n190 = Index Array(array=w598, index (row)=0) -> (element=w584:dbl[])  [unwired: 1 in]
                  n191 = call-poly <vilib>:"Decimate (continuous).vi"("error in (no error)"=w580, "averaging"=TRUE, "decimating factor"=w586, "X"=w584) -> ("error out"=w581:errorcluster, "Decimated Array"=w583:dbl[])  [unwired: 6 in]
                  n192 = local read "DeltaTOutput"() -> (w596:dbl)
                  n193 = local read "Averaging"() -> (w582:T1)
                  n194 = Get Date/Time In Seconds() -> (seconds since 1Jan1904=w595:timestamp)
                  n195 = Bundle By Name("t0"=w595, "dt"=w596, "Y"=w583) -> (w594:waveform(dbl))  [unwired: 1 in]
                  n196 = call-poly <vilib>:"FFT Power Spectrum and PSD.vi"("averaging parameters"=w582, "error in (no error)"=w581, "time signal"=w594) -> ("error out"=w593:errorcluster, "Power Spectrum / PSD"=w573:cluster{"f0":dbl, "df":dbl, "magnitude":dbl[]})  [unwired: 5 in, 2 out]
                  n197 = Unbundle By Name(w593) -> ("status"=w592:bool)
                  n198 = local read "stop"() -> (w590:bool)
                  n199 = Unbundle(w573) -> ("f0"=w578:dbl, "df"=w575:dbl, "magnitude"=w574:dbl[])
                  n200 = Or(x=w592, y=w590) -> (x .or. y?=w591:bool)
                  n201 = Multiply(x=0.0, y=w574) -> (x*y=w576:dbl[])
                  n202 = local read "nPlotPerRun"() -> (w588:u64)
                  n203 = Build Array(w574, w576) -> (w577:dbl[][])
                  n204 = Bundle("f0"=w578, "df"=w575, w577) -> (w572:cluster{"f0":dbl, "df":dbl, dbl[][]})  [unwired: 1 in]
                  n205 = Less?(x=w589, y=w588) -> (x < y?=w587:bool)
                  n206 = case shown="True" w587 {
                    tunnel: w572 -> [_ w604]
                    frame False {
                    }
                    frame True {
                      n207 = local write "PSD Y"(w604) -> ()
                    }
                  }
                }
                n208 = while {
                  tunnel: w542 -> [w655]
                  tunnel: w546 -> [w651]
                  stop <- w647 stop-if-true
                  # "Driving Array"
                  # "Generate Driving Array"
                  n209 = local read "fSampleAcquire"() -> (w662:dbl)
                  n210 = local read "PlotPoints"() -> (w661:u32)
                  n211 = local read "High Pass IIR filter specs"() -> (w657:T2)
                  n212 = Bundle("fSampleAcquire"=w662, "PlotPoints"=w661) -> (w663:cluster{"fSampleAcquire":dbl, "PlotPoints":u32})  [unwired: 1 in]
                  n213 = call <vilib>:"Uniform White Noise Waveform.vi"("sampling info"=w663) -> ("error out"=w673:errorcluster, "signal out"=w672:waveform(dbl))  [unwired: 9 in]
                  n214 = call-poly <vilib>:"Digital IIR Filter.vi"("IIR filter specifications"=w657, "error in (no error)"=w673, "signal in"=w672) -> ("error out"=w671:errorcluster, "signal out"=w670:waveform(dbl))  [unwired: 6 in, 1 out]
                  n215 = call <vilib>:"Normalize Waveform.vi"("error in (no error)"=w671, "waveform in"=w670) -> ("error out"=w669:errorcluster, "normalized waveform"=w668:waveform(dbl))  [unwired: 6 in, 2 out]
                  n216 = call <vilib>:"Waveform Scale and Offset.vi"("error in (no error)"=w669, "scale"="Ampl. (V)", "offset"="Offset (V)", "waveform in"=w668) -> ("error out"=w650:errorcluster, "waveform out"=w664:waveform(dbl))  [unwired: 6 in]
                  n217 = local read "nBufferPerPlot"() -> (w660:u32)
                  n218 = local read "BufferPoints"() -> (w659:u32)
                  n219 = Unbundle By Name(w664) -> ("Y"=w665:dbl[])
                  n220 = Merge Errors(w651, w650) -> (w652:errorcluster)
                  n221 = Build Array(w665) -> (w674:dbl[][])
                  n222 = Reshape Array(w674, w660, w659) -> (w658:dbl[][])
                  n223 = local read "PlotPeriod"() -> (w653:dbl)
                  n224 = Enqueue Element(queue=w655, element=w658, error in (no error)=w652) -> (error out=w649:errorcluster)  [unwired: 1 in, 2 out]
                  n225 = Multiply(x=100.0, y=w653) -> (x*y=w656:dbl)
                  n226 = Unbundle By Name(w649) -> ("status"=w648:bool)
                  n227 = local read "stop"() -> (w646:bool)
                  n228 = Wait (ms)(milliseconds to wait=w656) -> ()  [unwired: 1 out]
                  n229 = Or(x=w648, y=w646) -> (x .or. y?=w647:bool)
                }
                n230 = while {
                  tunnel: w542 -> [w681]
                  tunnel: w546 -> [w680]
                  tunnel: [w676] -> w537
                  tunnel: [w675] -> w539
                  stop <- w678 stop-if-true
                  # "Drive Queue Element Check"
                  n231 = Get Queue Status(queue=w681, error in (no error)=w680) -> (queue out=w675:refnum<queue>, error out=w676:errorcluster, # elements in queue=→"# Elements Drive Queue":i32)  [unwired: 1 in, 5 out]
                  n232 = Unbundle By Name(w676) -> ("status"=w679:bool)
                  n233 = local read "stop"() -> (w677:bool)
                  n234 = Or(x=w679, y=w677) -> (x .or. y?=w678:bool)
                  n235 = Wait (ms)(milliseconds to wait=100) -> ()  [unwired: 1 out]
                }
                n236 = for {
                  N: w554 -> [_]
                  tunnel: w542 -> [w626]
                  tunnel: w546 -> [w625]
                  tunnel: w548 -> [w628]
                  tunnel: [w630] -> w552
                  tunnel: w547 -> [w627]
                  tunnel: [w629] -> w553
                  tunnel: w545 -> [w621]
                  tunnel: w544 -> [w620]
                  tunnel: [w619] -> w534
                  tunnel: [w618] -> w532
                  i -> [w615]
                  stop <- w622 stop-if-true
                  # "Zero the first write segment and record PSD.  Then subtract his PSD. background from  new data PSDs."
                  # "Write Output to Drive Exciter"
                  n237 = Dequeue Element(queue=w626, error in (no error)=w625) -> (element=w613:dbl[][], error out=w624:errorcluster)  [unwired: 1 in, 2 out]
                  n238 = Equal To 0?(x=w615) -> (x = 0?=w614:bool)
                  n239 = case shown="True" w614 {
                    tunnel: w613 -> [w631 w634]
                    tunnel: [w631 w632] -> w612
                    frame False {
                    }
                    frame True {
                      n240 = Multiply(x=0.0, y=w634) -> (x*y=w632:dbl[][])
                    }
                  }
                  n241 = for {
                    tunnel: w628 -> [w635]
                    tunnel: w627 -> [w638]
                    tunnel: [w640] -> w630
                    tunnel: [w639] -> w629
                    tunnel: w612 -> [w642] mode=indexing
                    stop <- w644 stop-if-true
                    n242 = Build Array(w642) -> (w636:dbl[][])
                    n243 = local read "BufferPeriod"() -> (w643:dbl)
                    n244 = call-poly <vilib>:"DAQmx Write.vi"("task/channels in"=w635, "data"=w636, "timeout"=10.0, "error in"=w638) -> ("task out"=w640:refnum<k21>, "error out"=w639:errorcluster)  [unwired: 9 in, 1 out]
                    n245 = Unbundle By Name(w639) -> ("status"=w645:bool)
                    n246 = local read "stop"() -> (w641:bool)
                    n247 = Wait (ms)(milliseconds to wait=w643) -> ()  [unwired: 1 out]
                    n248 = Or(x=w645, y=w641) -> (x .or. y?=w644:bool)
                  }
                  n249 = Send Notification(notification=w612, notifier=w621, error in (no error)=w620) -> (notifier out=w618:refnum<notifier>, error out=w619:errorcluster)
                  n250 = Merge Errors(w629, w624, w619) -> (w623:errorcluster)
                  n251 = Unbundle By Name(w623) -> ("status"=w617:bool)
                  n252 = local read "stop"() -> (w616:bool)
                  n253 = Or(x=w616, y=w617) -> (x .or. y?=w622:bool)
                }
                n254 = local read "ReZero"() -> (w551:dbl[][])
                n255 = for {
                  tunnel: w551 -> [w610] mode=indexing
                  tunnel: w553 -> [w609]
                  tunnel: w552 -> [w607]
                  tunnel: [w606] -> w550
                  tunnel: [w605] -> w549
                  n256 = local read "BufferPeriod"() -> (w611:dbl)
                  n257 = Build Array(w610) -> (w608:dbl[][])
                  n258 = call-poly <vilib>:"DAQmx Write.vi"("task/channels in"=w607, "data"=w608, "error in"=w609) -> ("task out"=w606:refnum<k21>, "error out"=w605:errorcluster)  [unwired: 10 in, 1 out]
                  n259 = Wait (ms)(milliseconds to wait=w611) -> ()  [unwired: 1 out]
                }
                n260 = flat-sequence {
                  tunnel: w550 -> [w559]
                  tunnel: w549 -> [w558]
                  tunnel: [w555] -> w540
                  tunnel: w539 -> [w563]
                  tunnel: [w563] -> w538
                  tunnel: w537 -> [w562]
                  tunnel: [w562] -> w536
                  tunnel: [w561] -> w535
                  tunnel: w534 -> [w561]
                  tunnel: [w560] -> w533
                  tunnel: w532 -> [w560]
                  tunnel: [w567] -> w541
                  tunnel: w540 -> [w565]
                  tunnel: w538 -> [w571]
                  tunnel: w536 -> [w570]
                  tunnel: w535 -> [w569]
                  tunnel: w533 -> [w568]
                  frame #0 {
                    n261 = call <vilib>:"DAQmx Stop Task.vi"("task/channels in"=w559, "error in"=w558) -> ("task out"=w557:refnum<k21>, "error out"=w556:errorcluster)  [unwired: 12 in]
                    n262 = call <vilib>:"DAQmx Clear Task.vi"("task in"=w557, "error in"=w556) -> ("error out"=w555:errorcluster)  [unwired: 13 in]
                  }
                  frame #1 {
                    n263 = Release Queue(queue=w571, error in (no error)=w570) -> (error out=w564:errorcluster)  [unwired: 1 in, 2 out]
                    n264 = Release Notifier(notifier=w568, error in (no error)=w569) -> (error out=w566:errorcluster)  [unwired: 1 in, 2 out]
                    n265 = Merge Errors(w564, w565, w566) -> (w567:errorcluster)
                  }
                }
                n266 = call <vilib>:"Simple Error Handler.vi"("type of dialog (OK msg:1)"=w543, "error in (no error)"=w541) -> ()  [unwired: 3 in, 5 out]
              }
            }
            n267 = local write "stop"(w187) -> ()
            n268 = Open/Create/Replace File(file path (use dialog)=w192, operation (0:open)=T5."create", access (0:read/write)=enum16{"read/write", "read-only", "write-only"}."write-only") -> (refnum out=w155:refnum<file>, error out=w205:errorcluster)  [unwired: 1 in, 3 out]
            n269 = call <vilib>:"DAQmx Start Task.vi"("task/channels in"=w130, "error in"=w129) -> ("task out"=w127:refnum<k21>, "error out"=w128:errorcluster)  [unwired: 12 in]
            n270 = Refnum to Path(1:w155) -> (0:→"PathAtOpen":path)
            n271 = Write to Text File(file (use dialog)=w155, text=w202, error in=w205) -> (refnum out=w178:refnum<file>)  [unwired: 3 out]
            n272 = local read "nPlotPerRun"() -> (w200:u64)
            n273 = while {
              tunnel: w152 -> [w363]
              tunnel: w151 -> [w362]
              i -> [w330]
              stop <- w364 stop-if-true
              w344 = -0.9033  # CY1
              w345 = 0.1954  # CY2
              w346 = 0.2371  # CX2
              w347 = -0.8847  # CX1
              # "Y"
              # "X"
              # "Plot Data"
              n274 = Wait on Notification(notifier=w363, error in (no error)=w362) -> (notification=w367:dbl[][], error out=w366:errorcluster)  [unwired: 2 in, 2 out]
              n275 = Transpose 2D Array(2D array=w367) -> (transposed array=w378:dbl[][])
              n276 = Index Array(array=w378, index (row) #1=1, index (row) #2=2, index (row) #3=3) -> (element #1=w373:dbl[], element #2=w371:dbl[], element #3=w372:dbl[])  [unwired: 3 in]
              n277 = Divide(x=w373, y=w372) -> (x/y=w349:dbl[])
              n278 = Divide(x=w371, y=w372) -> (x/y=w350:dbl[])
              n279 = property on="Unit" class="Ring (strict)"() -> ("Value"=w342:u16)  [unwired: 2 in, 2 out]
              n280 = Multiply(x="LeverArm (m)", y=1000.0) -> (x*y=w337:dbl)
              n281 = case shown="0, Default" w342 {
                selector: w342 -> [w399 w402 w428 w454]
                tunnel: w350 -> [w400 w425 w452 w469]
                tunnel: w349 -> [w401 w411 w450 w467]
                tunnel: [w400 w417 w451 w468] -> w348
                tunnel: [w401 w408 w426 w459] -> w335
                tunnel: w347 -> [_ w407 w449 w466]
                tunnel: w346 -> [_ w406 w448 w465]
                tunnel: w345 -> [_ w405 w427 w464]
                tunnel: w337 -> [_ w404 w447 w463]
                tunnel: w344 -> [_ w403 w446 w462]
                frame 0, Default {
                  n282 = local write "PlotUnitIndex"(w399) -> ()
                }
                frame 1 {
                  n283 = Divide(x=w411, y=w407) -> (x/y=w416:dbl[])
                  n284 = Divide(x=w406, y=w404) -> (x/y=w409:dbl)
                  n285 = Divide(x=w405, y=w404) -> (x/y=w418:dbl)
                  n286 = Divide(x=w425, y=w403) -> (x/y=w424:dbl[])
                  n287 = local write "PlotUnitIndex"(w402) -> ()
                  n288 = Increment(x=w416) -> (x+1=w413:dbl[])
                  n289 = Decrement(x=w416) -> (x-1=w415:dbl[])
                  n290 = Increment(x=w424) -> (x+1=w421:dbl[])
                  n291 = Decrement(x=w424) -> (x-1=w423:dbl[])
                  n292 = Negate(x=w415) -> (-x=w414:dbl[])
                  n293 = Negate(x=w423) -> (-x=w422:dbl[])
                  n294 = Divide(x=w421, y=w422) -> (x/y=w420:dbl[])
                  n295 = Divide(x=w413, y=w414) -> (x/y=w412:dbl[])
                  n296 = Natural Logarithm(1:w420) -> (0:w419:dbl[])
                  n297 = Natural Logarithm(1:w412) -> (0:w410:dbl[])
                  n298 = Multiply(x=w410, y=w409) -> (x*y=w408:dbl[])
                  n299 = Multiply(x=w418, y=w419) -> (x*y=w417:dbl[])
                }
                frame 2 {
                  w436 = 2.0
                  n300 = Divide(x=w452, y=w446) -> (x/y=w431:dbl[])
                  n301 = Divide(x=w450, y=w449) -> (x/y=w441:dbl[])
                  n302 = Square(x=w431) -> (x^2=w435:dbl[])
                  n303 = Divide(x=w448, y=w447) -> (x/y=w440:dbl)
                  n304 = Divide(x=w427, y=w447) -> (x/y=w437:dbl)
                  n305 = Square(x=w441) -> (x^2=w445:dbl[])
                  n306 = Divide(x=w435, y=3.0) -> (x/y=w433:dbl[])
                  n307 = Divide(x=w445, y=3.0) -> (x/y=w443:dbl[])
                  n308 = Multiply(x=w440, y=w436) -> (x*y=w439:dbl)
                  n309 = Multiply(x=w436, y=w437) -> (x*y=w429:dbl)
                  n310 = Increment(x=w433) -> (x+1=w432:dbl[])
                  n311 = Increment(x=w443) -> (x+1=w442:dbl[])
                  n312 = Multiply(x=w432, y=w431) -> (x*y=w430:dbl[])
                  n313 = Multiply(x=w442, y=w441) -> (x*y=w438:dbl[])
                  n314 = Multiply(x=w429, y=w430) -> (x*y=w451:dbl[])
                  n315 = Multiply(x=w438, y=w439) -> (x*y=w426:dbl[])
                  "PlotUnitIndex" <- w428
                }
                frame 3 {
                  w457 = 2.0
                  n316 = local write "PlotUnitIndex"(w454) -> ()
                  n317 = Divide(x=w467, y=w466) -> (x/y=w455:dbl[])
                  n318 = Divide(x=w469, y=w462) -> (x/y=w453:dbl[])
                  n319 = Divide(x=w465, y=w463) -> (x/y=w461:dbl)
                  n320 = Divide(x=w464, y=w463) -> (x/y=w458:dbl)
                  n321 = Multiply(x=w461, y=w457) -> (x*y=w460:dbl)
                  n322 = Multiply(x=w457, y=w458) -> (x*y=w456:dbl)
                  n323 = Multiply(x=w455, y=w460) -> (x*y=w459:dbl[])
                  n324 = Multiply(x=w456, y=w453) -> (x*y=w468:dbl[])
                }
              }
              n325 = local read "DeltaTOutput"() -> (w376:dbl)
              n326 = Array Size(array=w335) -> (size(s)=→"SizeTimeSeries":i32)
              n327 = Get Date/Time In Seconds() -> (seconds since 1Jan1904=w377:timestamp)
              n328 = Bundle By Name("t0"=w377, "dt"=w376, "Y"=w348) -> (w375:waveform(dbl))  [unwired: 1 out]
              n329 = Bundle By Name("t0"=w377, "dt"=w376, "Y"=w335) -> (w374:waveform(dbl))  [unwired: 1 out]
              n330 = property on="Type" class="Ring (strict)"() -> ("Value"=w343:u16)  [unwired: 2 in, 2 out]
              n331 = call-poly <vilib>:"FFT Power Spectrum and PSD.vi"("export mode"=w343, "averaging parameters"="Averaging", "time signal"=w375) -> ("error out"=w379:errorcluster, "Power Spectrum / PSD"=w359:cluster{"f0":dbl, "df":dbl, "magnitude":dbl[]})  [unwired: 5 in, 2 out]
              n332 = call-poly <vilib>:"FFT Power Spectrum and PSD.vi"("export mode"=w343, "averaging parameters"="Averaging", "time signal"=w374) -> ("error out"=w380:errorcluster, "averages completed"=→"NAve":dbl, "Power Spectrum / PSD"=w360:cluster{"f0":dbl, "df":dbl, "magnitude":dbl[]})  [unwired: 5 in, 1 out]
              n333 = Merge Errors(w380, w379, w366) -> (w365:errorcluster)
              n334 = Unbundle By Name(w360) -> ("f0"=w354:dbl, "df"=w336:dbl, "magnitude"=w341:dbl[])
              "df" <- w336
              n335 = Unbundle By Name(w359) -> ("magnitude"=w340:dbl[])  [unwired: 2 out]
              n336 = Unbundle By Name(w365) -> ("status"=w357:bool)
              n337 = local read "stop"() -> (w356:bool)
              n338 = Square Root(x=w341) -> (sqrt(x)=w327:dbl[])
              n339 = Square Root(x=w340) -> (sqrt(x)=w328:dbl[])
              n340 = Or(x=w356, y=w357) -> (x .or. y?=w364:bool)
              n341 = Equal To 0?(x=w330) -> (x = 0?=w329:bool)
              n342 = case shown="True" w329 {
                tunnel: w328 -> [_ w398]
                tunnel: w327 -> [_ w389]
                frame False {
                }
                frame True {
                  n343 = Array Max & Min(array=w398) -> (max value=w395:dbl, min value=w390:dbl)  [unwired: 2 out]
                  n344 = Array Max & Min(array=w389) -> (max value=w388:dbl, min value=w383:dbl)  [unwired: 2 out]
                  n345 = Logarithm Base 10(1:w395) -> (0:w394:dbl)
                  n346 = Logarithm Base 10(1:w388) -> (0:w387:dbl)
                  n347 = Round Toward +Infinity(x=w394) -> (ceil(x): smallest int >= x=w393:dbl)
                  n348 = Round Toward +Infinity(x=w387) -> (ceil(x): smallest int >= x=w386:dbl)
                  n349 = Power Of 10(x=w393) -> (10^x=w391:dbl)
                  n350 = Power Of 10(x=w386) -> (10^x=w381:dbl)
                  n351 = property on="PSD Y" class="WFGraph (strict)"("YScale.Maximum"=w391) -> ()  [unwired: 2 in, 2 out]
                  n352 = property on="PSD X" class="WFGraph (strict)"("YScale.Maximum"=w381) -> ()  [unwired: 2 in, 2 out]
                  n353 = Logarithm Base 10(1:w390) -> (0:w397:dbl)
                  n354 = Logarithm Base 10(1:w383) -> (0:w385:dbl)
                  n355 = Round Toward -Infinity(1:w397) -> (0:w396:dbl)
                  n356 = Round Toward -Infinity(1:w385) -> (0:w384:dbl)
                  n357 = Power Of 10(x=w396) -> (10^x=w392:dbl)
                  n358 = Power Of 10(x=w384) -> (10^x=w382:dbl)
                  n359 = property on="PSD Y" class="WFGraph (strict)"("YScale.Minimum"=w392) -> ()  [unwired: 2 in, 2 out]
                  n360 = property on="PSD X" class="WFGraph (strict)"("YScale.Minimum"=w382) -> ()  [unwired: 2 in, 2 out]
                }
              }
              n361 = Build Array(w327, w328) -> (w332:dbl[][])
              n362 = Build Array(w328, w327) -> (w331:dbl[][])
              n363 = Bundle("f0"=w354, "df"=w336, w331) -> (w351:cluster{"f0":dbl, "df":dbl, dbl[][]})  [unwired: 1 in]
              n364 = Bundle("f0"=w354, "df"=w336, w332) -> (w352:cluster{"f0":dbl, "df":dbl, dbl[][]})  [unwired: 1 in]
              n365 = Bundle("f0"=w354, "df"=w336, w332) -> (w353:cluster{"f0":dbl, "df":dbl, dbl[][]})  [unwired: 1 in]
              n366 = local read "nPlotPerRun"() -> (w355:u64)
              n367 = Less?(x=w330, y=w355) -> (x < y?=w361:bool)
              n368 = case shown="True" w361 {
                tunnel: w353 -> [_ w470]
                tunnel: w352 -> [_ w472]
                tunnel: w351 -> [_ w471]
                frame False {
                }
                frame True {
                  n369 = local write "Plot1"(w470) -> ()
                  n370 = local write "Plot2"(w470) -> ()
                  n371 = local write "Plot3"(w470) -> ()
                  n372 = local write "Plot4"(w470) -> ()
                  n373 = local read "Excite"() -> (w473:bool)
                  n374 = local write "Plot5"(w470) -> ()
                  n375 = local write "Plot6"(w470) -> ()
                  n376 = local write "Plot7"(w470) -> ()
                  n377 = local write "Plot8"(w470) -> ()
                  n378 = case shown="False" w473 {
                    tunnel: w472 -> [w474 w476]
                    tunnel: w471 -> [w475 _]
                    frame False {
                      n379 = local write "PSD Y"(w475) -> ()
                      n380 = property on="PSD X" class="WFGraph (strict)"("Val(Sgnl)"=w474) -> ()  [unwired: 2 in, 2 out]
                    }
                    frame True {
                      n381 = local write "PSD X"(w476) -> ()
                    }
                  }
                }
              }
              "Plot" <- w330
            }
            n382 = while {
              tunnel: w178 -> [w242]
              tunnel: w152 -> [w239]
              tunnel: w151 -> [w238]
              tunnel: w154 -> [w237]
              tunnel: w153 -> [w236]
              i -> [w220]
              stop <- w240 stop-if-true
              # "DATA\nTime\nX\nY\nSUM"
              # "Write to Temp/Data File"
              n383 = Dequeue Element(queue=w237, error in (no error)=w236) -> (element=w224:dbl[][], error out=w226:errorcluster)  [unwired: 1 in, 2 out]
              n384 = local read "Input Data Type"() -> (w227:u16)
              n385 = Array Size(array=w224) -> (size(s)=→"Raw Data Size":i32[])
              n386 = case shown="2" w227 {
                tunnel: w226 -> [w246 w271 w291]
                tunnel: w224 -> [w245 w274 w294]
                tunnel: [w246 w271 w291] -> w225
                tunnel: [w245 w269 w289] -> w221
                frame 0, Default {
                }
                frame 1 {
                  # "Time\nQ 1+/-  —  4+/-"
                  # "Time\nX\nY\nSUM"
                  n387 = Index Array(array=w274, index (col) #1=0, index (col) #2=1, index (col) #3=2, index (col) #4=3, index (col) #5=4, index (col) #6=5, index (col) #7=6, index (col) #8=7, index (col) #9=8) -> (element #1=w272:dbl[], element #2=w258:dbl[], element #3=w257:dbl[], element #4=w256:dbl[], element #5=w255:dbl[], element #6=w254:dbl[], element #7=w253:dbl[], element #8=w260:dbl[], element #9=w259:dbl[])  [unwired: 9 in]
                  n388 = Subtract(x=w258, y=w257) -> (x-y=w251:dbl[])
                  n389 = Subtract(x=w256, y=w255) -> (x-y=w250:dbl[])
                  n390 = Subtract(x=w254, y=w253) -> (x-y=w252:dbl[])
                  n391 = Subtract(x=w260, y=w259) -> (x-y=w249:dbl[])
                  n392 = Subtract(x=w251, y=w250) -> (x-y=w247:dbl[])
                  n393 = Subtract(x=w252, y=w249) -> (x-y=w248:dbl[])
                  n394 = Compound Arithmetic op=ADD(w251, w250, w252, w249) -> (w265:dbl[])
                  n395 = Add(x=w247, y=w248) -> (x+y=w268:dbl[])
                  n396 = Subtract(x=w247, y=w248) -> (x-y=w267:dbl[])
                  n397 = Negate(x=w268) -> (-x=w266:dbl[])
                  n398 = Build Array(w272, w267, w266, w265) -> (w270:dbl[][])
                  n399 = Transpose 2D Array(2D array=w270) -> (transposed array=w269:dbl[][])
                }
                frame 2 {
                  # "Time\nQ 1 —  4"
                  # "Time\nX\nY\nSUM"
                  n400 = Index Array(array=w294, index (col) #1=0, index (col) #2=1, index (col) #3=2, index (col) #4=3, index (col) #5=4) -> (element #1=w292:dbl[], element #2=w282:dbl[], element #3=w281:dbl[], element #4=w280:dbl[], element #5=w279:dbl[])  [unwired: 5 in]
                  n401 = Subtract(x=w282, y=w281) -> (x-y=w283:dbl[])
                  n402 = Subtract(x=w280, y=w279) -> (x-y=w284:dbl[])
                  n403 = Compound Arithmetic op=ADD(w282, w281, w280, w279) -> (w285:dbl[])
                  n404 = Add(x=w283, y=w284) -> (x+y=w288:dbl[])
                  n405 = Subtract(x=w283, y=w284) -> (x-y=w287:dbl[])
                  n406 = Negate(x=w288) -> (-x=w286:dbl[])
                  n407 = Build Array(w292, w287, w286, w285) -> (w290:dbl[][])
                  n408 = Transpose 2D Array(2D array=w290) -> (transposed array=w289:dbl[][])
                }
              }
              n409 = Array Size(array=w221) -> (size(s)=→"Converted Data Size":i32[])
              n410 = local read "Oversample"() -> (w228:bool)
              n411 = Equal To 0?(x=w220) -> (x = 0?=w219:bool)
              n412 = case shown="True" w228 {
                tunnel: w221 -> [w300 w308]
                tunnel: [w300 w306] -> w232
                tunnel: [w299 w303] -> w230
                tunnel: w225 -> [w299 w304]
                tunnel: w219 -> [_ w301]
                frame False {
                }
                frame True {
                  w316 = TRUE
                  n413 = local read "DecimFactor"() -> (w317:u32)
                  n414 = Index Array(array=w308, index (col) #1=0, index (col) #2=1, index (col) #3=2, index (col) #4=3) -> (element #1=w320:dbl[], element #2=w302:dbl[], element #3=w319:dbl[], element #4=w318:dbl[])  [unwired: 4 in]
                  n415 = call-poly <vilib>:"Decimate (continuous).vi"("reset"=w301, "averaging"=w316, "decimating factor"=w317, "X"=w302) -> ("error out"=w311:errorcluster, "Decimated Array"=w305:dbl[])  [unwired: 6 in]
                  n416 = call-poly <vilib>:"Decimate (continuous).vi"("reset"=w301, "averaging"=w316, "decimating factor"=w317, "X"=w319) -> ("error out"=w309:errorcluster, "Decimated Array"=w314:dbl[])  [unwired: 6 in]
                  n417 = call-poly <vilib>:"Decimate (continuous).vi"("reset"=w301, "averaging"=w316, "decimating factor"=w317, "X"=w318) -> ("error out"=w312:errorcluster, "Decimated Array"=w313:dbl[])  [unwired: 6 in]
                  n418 = call-poly <vilib>:"Decimate (continuous).vi"("reset"=w301, "averaging"=w316, "decimating factor"=w317, "X"=w320) -> ("error out"=w310:errorcluster, "Decimated Array"=w315:dbl[])  [unwired: 6 in]
                  n419 = Build Array(w315, w305, w314, w313) -> (w307:dbl[][])
                  n420 = Merge Errors(w310, w311, w309, w312, w304) -> (w303:errorcluster)
                  n421 = Transpose 2D Array(2D array=w307) -> (transposed array=w306:dbl[][])
                }
              }
              n422 = local read "nPlotPerRun"() -> (w234:u64)
              "WriteLimit" <- w234
              n423 = Send Notification(notification=w232, notifier=w239, error in (no error)=w238) -> (error out=w229:errorcluster)  [unwired: 1 out]
              n424 = Array To Spreadsheet String(array=w232, 3:"%.6f") -> (spreadsheet string=w243:string)  [unwired: 1 in]
              n425 = Merge Errors(w230, w229) -> (w231:errorcluster)
              n426 = Less?(x=w220, y=w234) -> (x < y?=w233:bool)
              n427 = case shown="True" w233 {
                tunnel: w243 -> [_ w326]
                tunnel: w242 -> [_ w325]
                frame False {
                }
                frame True {
                  n428 = Write to Text File(file (use dialog)=w325, text=w326) -> ()  [unwired: 2 in, 3 out]
                }
              }
              n429 = Unbundle By Name(w231) -> ("status"=w241:bool)
              n430 = local read "stop"() -> (w235:bool)
              n431 = Or(x=w241, y=w235) -> (x .or. y?=w240:bool)
              "WriteNumber" <- w220
            }
            n432 = while {
              tunnel: w154 -> [w856]
              tunnel: w153 -> [w855]
              stop <- w852 stop-if-true
              # "Response Queue Element Check"
              n433 = Get Queue Status(queue=w856, error in (no error)=w855) -> (error out=w851:errorcluster, # elements in queue=→"# Elements Response Queue":i32)  [unwired: 1 in, 6 out]
              n434 = Unbundle By Name(w851) -> ("status"=w854:bool)
              n435 = local read "stop"() -> (w853:bool)
              n436 = Or(x=w853, y=w854) -> (x .or. y?=w852:bool)
              n437 = Wait (ms)(milliseconds to wait=100) -> ()  [unwired: 1 out]
            }
            n438 = for {
              N: w200 -> [_]
              tunnel: w127 -> [w824]
              tunnel: [w825] -> w190
              tunnel: w128 -> [w823]
              tunnel: [w817] -> w189
              tunnel: w154 -> [w811]
              tunnel: w153 -> [w810]
              i -> [w815]
              stop <- w813 stop-if-true
              # "Read Sample Data"
              n439 = local read "PlotPeriod"() -> (w816:dbl)
              n440 = local read "nBufferPerPlot"() -> (w820:u32)
              n441 = Multiply(x=w815, y=w816) -> (x*y=w814:dbl)
              n442 = for {
                N: w820 -> [_]
                shift-right: [w830] -> w825
                shift-left: w824 -> [w831]
                shift-right: [w829] -> w817
                shift-left: w823 -> [w832]
                tunnel: [w843] -> w819 mode=concatenating
                tunnel: w814 -> [w838]
                i -> [w841]
                stop <- w844 stop-if-true
                n443 = local read "BufferPeriod"() -> (w842:dbl)
                n444 = local read "BufferPoints"() -> (w827:u32)
                n445 = local read "time vector"() -> (w837:dbl[])
                n446 = Multiply(x=w841, y=w842) -> (x*y=w840:dbl)
                n447 = call-poly <vilib>:"DAQmx Read.vi"("task/channels in"=w831, "number of samples per channel"=w827, "timeout"=10.0, "error in"=w832) -> ("task out"=w830:refnum<k21>, "data"=w828:dbl[][], "error out"=w829:errorcluster)  [unwired: 9 in]
                n448 = Add(x=w840, y=w838) -> (x+y=w834:dbl)
                n449 = Add(x=w834, y=w837) -> (x+y=w836:dbl[])
                n450 = Greater Than 0?(x=w834) -> (x > 0?=w835:bool)
                n451 = Unbundle By Name(w829) -> ("status"=w845:bool)
                n452 = case shown="True" w835 {
                  tunnel: w834 -> [_ w850]
                  frame False {
                  }
                  frame True {
                    n453 = local read "RunPeriod"() -> (w847:dbl)
                    n454 = Multiply(x=w850, y=100) -> (x*y=w846:dbl)
                    n455 = Divide(x=w846, y=w847) -> (x/y=→"Progress":dbl)
                  }
                }
                n456 = Build Array (concatenate)(w836, w828) -> (w839:dbl[][])
                n457 = local read "stop"() -> (w833:bool)
                n458 = Transpose 2D Array(2D array=w839) -> (transposed array=w843:dbl[][])
                n459 = Or(x=w845, y=w833) -> (x .or. y?=w844:bool)
              }
              n460 = Enqueue Element(queue=w811, element=w819, error in (no error)=w810) -> (error out=w818:errorcluster)  [unwired: 1 in, 2 out]
              n461 = Merge Errors(w817, w818) -> (w822:errorcluster)
              n462 = Unbundle By Name(w822) -> ("status"=w821:bool)
              n463 = local read "stop"() -> (w812:bool)
              n464 = Or(x=w821, y=w812) -> (x .or. y?=w813:bool)
            }
            n465 = flat-sequence {
              tunnel: [w722] -> w191
              tunnel: w190 -> [w726]
              tunnel: w189 -> [w725]
              tunnel: w155 -> [w727]
              tunnel: [w727] -> w175
              tunnel: w191 -> [w734]
              tunnel: [w734] -> w188
              tunnel: [w733] -> w176
              tunnel: w175 -> [w733]
              tunnel: w188 -> [w740]
              tunnel: [w740] -> w180
              tunnel: [w739] -> w177
              tunnel: w176 -> [w739]
              tunnel: w180 -> [w741]
              tunnel: w177 -> [w758]
              tunnel: [w757] -> w150
              tunnel: w150 -> [w764]
              tunnel: [w760] -> w147
              tunnel: [w759] -> w148
              frame #0 {
                n466 = Refnum to Path(1:w727) -> (0:→"PathAtClose":path)
                n467 = call <vilib>:"DAQmx Stop Task.vi"("task/channels in"=w726, "error in"=w725) -> ("task out"=w724:refnum<k21>, "error out"=w723:errorcluster)  [unwired: 12 in]
                n468 = Wait (ms)(milliseconds to wait=1000) -> ()  [unwired: 1 out]
                n469 = call <vilib>:"DAQmx Clear Task.vi"("task in"=w724, "error in"=w723) -> ("error out"=w722:errorcluster)  [unwired: 13 in]
                "Step" <- 1
              }
              frame #1 {
                n470 = local write "Step"(2) -> ()
                n471 = local write "stop"(TRUE) -> ()
              }
              frame #2 {
                n472 = local read "PlotPeriod"() -> (w736:dbl)
                n473 = local write "Step"(3) -> ()
                n474 = Multiply(x=w736, y=1000) -> (x*y=w735:dbl)
                n475 = Wait (ms)(milliseconds to wait=w735) -> ()  [unwired: 1 out]
              }
              frame #3 {
                w744 = TRUE
                n476 = local write "Step"(4) -> ()
                n477 = Initialize Array(0.0, 1, 3) -> (w754:dbl[][])
                n478 = Close File(refnum=w758, error in=w741) -> (error out=w756:errorcluster)  [unwired: 1 out]
                n479 = Obtain Queue(name (unnamed)="Response Queue", element data type=w754) -> (queue out=w751:refnum<queue>, error out=w753:errorcluster)  [unwired: 3 in, 1 out]
                n480 = Obtain Notifier(name (unnamed)="Response Notifier", notification data type=w754) -> (notifier out=w750:refnum<notifier>, error out=w752:errorcluster)  [unwired: 2 in, 1 out]
                n481 = Release Queue(queue=w751, force destroy? (F)=w744, error in (no error)=w753) -> (error out=w743:errorcluster)  [unwired: 2 out]
                n482 = Release Notifier(notifier=w750, force destroy? (F)=w744, error in (no error)=w752) -> (error out=w742:errorcluster)  [unwired: 2 out]
                n483 = Merge Errors "Merge Errors"(w756, w743, w742) -> (w757:errorcluster)
              }
              frame #4 {
                w763 = T8 4 items=["no dialog", "OK message", "continue/stop", "OK + warnings", "cont./stop + warn"] ("type of dialog (OK msg:1)")
                n484 = local read "Excite"() -> (w766:bool)
                n485 = call <vilib>:"Simple Error Handler.vi"("type of dialog (OK msg:1)"=w763, "error in (no error)"=w764) -> ("error?"=w765:bool)  [unwired: 3 in, 4 out]
                n486 = local write "Step"(5) -> ()
                n487 = Or(x=w766, y=w765) -> (x .or. y?=w762:bool)
                n488 = case shown="False" w762 {
                  tunnel: [w769 2] -> w759
                  tunnel: [w768 FALSE] -> w760
                  frame False {
                    n489 = case shown="True" "AutoSave" {
                      tunnel: [0 w774] -> w769
                      tunnel: [FALSE w775] -> w768
                      frame False {
                        n490 = property on="Out" class="Path"("Val(Sgnl)"=path "") -> ()  [unwired: 2 in, 2 out]
                        n491 = property on="File" class="Str"("Val(Sgnl)"="") -> ()  [unwired: 2 in, 2 out]
                      }
                      frame True {
                        n492 = Format Into String(format string="\\n\\n%s\\n%s\\n%s", initial string="Check the parameters in the blue panel. ", "\"Save\" = Save immediately", "\"Change, then Save\" = Update Parameters, then press Save", "\"Cancel\" = Don't Save.") -> (resulting string=w777:string)  [unwired: 1 in, 1 out]
                        n493 = call <vilib>:"Three Button Dialog.vi"("Window Title (\"\")"="Parameter Check ", "Center Button Text (\"No\")"="Change, then Save", "Left Button Text (\"Yes\")"="Save", "message"=w777) -> ("Which Button?"=w776:T9)  [unwired: 2 in, 5 out]
                        n494 = case shown="\"Left Button\", Default" w776 {
                          tunnel: [FALSE FALSE FALSE FALSE] -> w775
                          tunnel: [2 0 2 2] -> w774
                          frame "Left Button", Default {
                            n495 = property on="Write Light" class="Bool (strict)"("Val(Sgnl)"=TRUE) -> ()  [unwired: 2 in, 2 out]
                            n496 = local write "WriteNewHeader"(FALSE) -> ()
                          }
                          frame "Center Button" {
                            n497 = property on="Out" class="Path"("Val(Sgnl)"=path "") -> ()  [unwired: 2 in, 2 out]
                            n498 = local write "WriteNewHeader"(TRUE) -> ()
                          }
                          frame "Right Button" {
                            # "\"Cancel\" = Don't Save."
                            n499 = local read "TempFilePath"() -> (w794:path)
                            n500 = local read "DataFilePath"() -> (w795:path)
                            n501 = property on="Out" class="Path"("Val(Sgnl)"=path "") -> ()  [unwired: 2 in, 2 out]
                            n502 = Move(source path=w795, 10:w794) -> ()  [unwired: 3 in, 3 out]
                          }
                          frame "Window Close" {
                            # "\"Cancel\" = Don't Save."
                            n503 = local read "TempFilePath"() -> (w800:path)
                            n504 = local read "DataFilePath"() -> (w799:path)
                            n505 = property on="Out" class="Path"("Val(Sgnl)"=path "") -> ()  [unwired: 2 in, 2 out]
                            n506 = Move(source path=w799, 10:w800) -> ()  [unwired: 3 in, 3 out]
                          }
                        }
                      }
                    }
                  }
                  frame True {
                    n507 = property on="Out" class="Path"("Val(Sgnl)"=path "") -> ()  [unwired: 2 in, 2 out]
                  }
                }
              }
            }
            n508 = Boolean To (0,1)(Boolean=w147) -> (0, 1=w149:i16)
            n509 = property on="Manual Save" class="Bool (strict)"("DisabledEnum"=w148) -> ()  [unwired: 2 in, 2 out]
            n510 = property on="RunLight" class="Bool (strict)"("Value"=w147) -> ()  [unwired: 2 in, 2 out]
            n511 = local write "stop"(w147) -> ()
            n512 = property on="Start" class="Bool (strict)"("Value"=w147) -> ()  [unwired: 2 in, 2 out]
            n513 = local write "Progress"(w149) -> ()
          }
          event "Offset (V)", "Ampl. (V)": Value Change {
            n514 = event-data() -> ()  [unwired: 7 out]
            n515 = local read "Ampl. (V)"() -> (w866:sgl)
            n516 = local read "Offset (V)"() -> (w865:sgl)
            n517 = Absolute Value(x=w865) -> (abs(x)=w862:sgl)
            n518 = Absolute Value(x=w866) -> (abs(x)=w860:sgl)
            n519 = Add(x=w862, y=w860) -> (x+y=w864:sgl)
            n520 = local read "Max Value"() -> (w861:dbl)
            n521 = Greater?(x=w864, y=w861) -> (0:w863:bool)
            n522 = Subtract(x=w861, y=w860) -> (x-y=w859:dbl)
            n523 = case shown="True" w863 {
              tunnel: w859 -> [_ w867]
              frame False {
              }
              frame True {
                n524 = local write "Offset (V)"(w867) -> ()
              }
            }
          }
          event "Averaging.weighting mode": Value Change {
            n525 = event-data() -> ()  [unwired: 7 out]
            n526 = property on="Averaging" class="Clust (strict)"() -> ("Value"=w873:T1)  [unwired: 2 in, 2 out]
            n527 = Unbundle By Name(w873) -> ("Averaging"=w872:T6, "weighting mode"=w868:enum16{"Linear", "Exponential"})  [unwired: 1 out]
            n528 = Equal To 0?(x=w868) -> (x = 0?=w870:bool)
            n529 = case shown="True" w870 {
              tunnel: [w874 w875] -> w869
              tunnel: w868 -> [w874 _]
              frame False {
              }
              frame True {
                n530 = property on="nPlotPerRun" class="DigNum (strict)"() -> ("Value"=w875:u64)  [unwired: 2 in, 2 out]
              }
            }
            n531 = Bundle("Averaging"=w872, "weighting mode"=w868, "Value"=w869) -> (w871:T10)  [unwired: 1 in]
            n532 = property on="Averaging" class="Clust (strict)"("Value"=w871) -> ()  [unwired: 2 in, 2 out]
          }
          event "Manual Save": Mouse Down; "Write Light": Value Change {
            n533 = event-data() -> ()  [unwired: 3 out]
            n534 = flat-sequence {
              frame #0 {
                n535 = local write "stop"(FALSE) -> ()
                "Location" <- "Start of \"Save\""
              }
              frame #1 {
                w891 = 10.0
                w892 = -10.0
                w889 = "MultiQ Data File:\\t%s \\n\\nSample Name:\\t%s \\nSample Label:\\t %s\\nDate:\\t%s \\nTime:\\t %s \\nWho:\\t%s \\nRun Number:\\t%d \\nDuration:\\t %.6f s \\nRate:\\t%7.2f Hz \\nData Points:\\t %d \\nRange:\\t(%5.1f, %5.1f) Volts\\nMin Frequency:\\t %9.2f kHz \\nPressure:\\t%9.2e torr\\nComment:\\t%s\\n\\n"  # MultiQ Data File:\t%s \n\nSample Name:\t%s \nSample Label:\t %s\nDate:\t%s \nTime:\t %s \nWho:\t%s \nRun Number:\t%d \nDuration:\t %.6f s \nRate:\t%7.2f Hz \nData Points:\t %d \nRange:\t(%5.1f, %5.1f) Volts\nMin Frequency:\t %9.2f kHz \nPressure:\t%9.2e torr\nComment:\t%s\n\n
                # "Make the HTML Table"
                # "Make the Data File Header"
                # "Date"
                # "Time"
                # "Write HTML Data in Table Row"
                # "HTML File Exists?"
                # "Update the Run Number"
                n536 = property on="Start Time" class="AbsTime (strict)"() -> ("Value"=w915:timestamp)  [unwired: 2 in, 2 out]
                n537 = local read "NDataPointsOutput"() -> (w893:u64)
                n538 = local read "fSampleOutput"() -> (w894:dbl)
                n539 = local read "RunPeriod"() -> (w895:dbl)
                n540 = local read "Run Number"() -> (w888:i8)
                n541 = local read "Comment"() -> (w878:string)
                n542 = local read "fMinPlot"() -> (w897:dbl)
                n543 = Format Date/Time String(time format string (%c)="%d %b %Y", seconds (now)=w915) -> (date/time string=w911:string)  [unwired: 1 out]
                n544 = Format Date/Time String(time format string (%c)="%H:%M:%S", seconds (now)=w915) -> (date/time string=w910:string)  [unwired: 1 out]
                n545 = Number To Decimal String(number="Run Number", width (-)=2) -> (decimal integer string=w927:string)
                n546 = Path To String(path="Path") -> (string=w919:string)
                n547 = Strip Path(path="Path") -> (stripped path=w922:path, name=w896:string)
                n548 = call <vilib>:"Trim Whitespace.vi"("string"=w927) -> ("trimmed string"=w916:string)  [unwired: 1 in]
                n549 = Format Into String(format string="<h2><b>Sample: </b>#%s,  %s </h2>", "Name", "Label") -> (resulting string=→"HTML \nTitle":string)  [unwired: 2 in, 1 out]
                n550 = Concatenate Strings(w896, "_", w916, ".txt") -> (w881:string)
                n551 = Concatenate Strings(w919, "_table.html") -> (w924:string)
                n552 = Build Path(base path=w922, name or relative path=w881) -> (appended path=w884:path)
                n553 = String To Path(string=w924) -> (path=w914:path)
                n554 = Format Into String(format string=w889, w881, "Name", "Label", w911, w910, "Who", w888, w895, w894, w893, w892, w891, w897, "Pressure (t)", w878) -> (resulting string=w903:string, error out=w904:errorcluster)  [unwired: 2 in]
                n555 = Format Into String(format string="<tr  align=\"center\" valign=\"middle\"> \\n <td>%s</td> <td>%s</td>  <td>%s</td> <td>%d</td>\n<td>%.6f</td> <td>%7.2f </td>\n<td>%d</td> <td>%5.1f</td>\n<td>%5.1f</td> <td>%9.2f</td> \n<td>%9.2e</td>\n<td>%s</td> <td>%s</td>\\n \n</tr>\\n\\n", error in=w904, w911, w910, "Who", w888, w895, w894, w893, w892, w891, w897, "Pressure (t)", w881, w878) -> (resulting string=w902:string, error out=w901:errorcluster)  [unwired: 1 in]
                n556 = local read "DataFilePath"() -> (w885:path)
                n557 = Equal?(x=w885, y=w884) -> (x = y?=w886:bool)
                n558 = local read "WriteNewHeader"() -> (w882:bool)
                n559 = case shown="False" w886 {
                  tunnel: w885 -> [w952 w953]
                  tunnel: w884 -> [w951 _]
                  tunnel: [w950 w953] -> w883
                  frame False {
                    n560 = Move(source path=w952, 10:w951) -> (3:w950:path)  [unwired: 3 in, 2 out]
                  }
                  frame True {
                  }
                }
                n561 = case shown="True" w882 {
                  tunnel: w903 -> [_ w944]
                  tunnel: w901 -> [w938 w943]
                  tunnel: [w938 w942] -> w900
                  tunnel: [w937 w941] -> w899
                  tunnel: w883 -> [w937 w939]
                  frame False {
                  }
                  frame True {
                    # "Open the Data File\nWrite Header"
                    n562 = Open/Create/Replace File(file path (use dialog)=w939, error in=w943, operation (0:open)=T5."open", access (0:read/write)=enum16{"read/write", "read-only", "write-only"}."write-only") -> (refnum out=w948:refnum<file>, error out=w947:errorcluster)  [unwired: 3 out]
                    n563 = Write to Text File(file (use dialog)=w948, text=w944, error in=w947) -> (refnum out=w940:refnum<file>, error out=w945:errorcluster)  [unwired: 2 out]
                    n564 = Close File(refnum=w940, error in=w945) -> (path=w941:path, error out=w942:errorcluster)
                  }
                }
                n565 = call <vilib>:"Check if File or Folder Exists.vi"("error in (no error)"=w900, "path"=w914) -> ("error out"=w931:errorcluster, "file or folder exists?"=w933:bool, "dup path"=w932:path)  [unwired: 7 out]
                n566 = case shown="False" w933 {
                  tunnel: w932 -> [w962 w969]
                  tunnel: w931 -> [w963 w968]
                  tunnel: [w959 w967] -> w930
                  tunnel: [w957 w966] -> w929
                  frame False {
                    # "Create File & Write Header Row"
                    n567 = Open/Create/Replace File(file path (use dialog)=w962, error in=w963, operation (0:open)=T5."create", access (0:read/write)=enum16{"read/write", "read-only", "write-only"}."write-only") -> (refnum out=w961:refnum<file>, error out=w960:errorcluster)  [unwired: 3 out]
                    n568 = property on="HTML \nTitle" class="Str"() -> ("Value"=w955:string)  [unwired: 2 in, 2 out]
                    n569 = Format Into String(format string="%s\\n%s\\n%s\\n\\n", initial string=w961, error in=w960, w955, "<table border=\"1\" cellspacing =\"1\" cellpadding=\"6\">", "<tr  align=\"center\" valign=\"middle\"> <th>Date</th> <th>Time</th> <th>Who</th><th>Run #</th> <th>Duration (s)</th> <th>Rate (Hz)</th> <th>N Points</th> <th>Min Value (V)</th> <th>Max Value (V)</th><th>Min Freq (jkHz)</th> <th>Pressure (torr)</th>  <th>Filename</th><th>Comment</th> </tr>") -> (resulting string=w959:refnum<file>, error out=w957:errorcluster)
                  }
                  frame True {
                    # "Open File and Go To End"
                    n570 = Open/Create/Replace File(file path (use dialog)=w969, error in=w968, operation (0:open)=T5."open", access (0:read/write)=enum16{"read/write", "read-only", "write-only"}."write-only") -> (refnum out=w973:refnum<file>, error out=w972:errorcluster)  [unwired: 3 out]
                    n571 = Set File Position(refnum=w973, from (0:start)=1, error in=w972) -> (refnum out=w967:refnum<file>, error out=w966:errorcluster)  [unwired: 1 out]
                  }
                }
                n572 = Write to Text File(file (use dialog)=w930, text=w902, error in=w929) -> (refnum out=w936:refnum<file>, error out=w935:errorcluster)  [unwired: 2 out]
                n573 = Close File(refnum=w936, error in=w935) -> (error out=w934:errorcluster)  [unwired: 1 out]
                n574 = call <vilib>:"Simple Error Handler.vi"("type of dialog (OK msg:1)"=3, "error in (no error)"=w934) -> ("error?"=w879:bool)  [unwired: 7 out]
                n575 = case shown="False" w879 {
                  tunnel: w899 -> [w978 _]
                  tunnel: [w978 path ""] -> w912
                  tunnel: [2 0] -> w880
                  frame False {
                    n576 = property on="Run Number" class="DigNum (strict)"() -> ("Value"=w975:i8)  [unwired: 2 in, 2 out]
                    n577 = Increment(x=w975) -> (x+1=w977:i8)
                    n578 = property on="Run Number" class="DigNum (strict)"("Val(Sgnl)"=w977) -> ()  [unwired: 2 in, 2 out]
                  }
                  frame True {
                  }
                }
                "Out" <- w912
                n579 = property on="Manual Save" class="Bool (strict)"("Val(Sgnl)"=w879) -> ()  [unwired: 2 in, 2 out]
                n580 = property on="Write Light" class="Bool (strict)"("Value"=w879) -> ()  [unwired: 2 in, 2 out]
                n581 = property on="Manual Save" class="Bool (strict)"("DisabledEnum"=w880) -> ()  [unwired: 2 in, 2 out]
                n582 = Strip Path(path=w912) -> (name=→"File":string)  [unwired: 1 out]
              }
              frame #2 {
                n583 = local write "Location"("End of \"Save\"") -> ()
              }
            }
          }
          event "Substrate", "Mode Scale", "Range (%)", "Sample Modes": Value Change {
            w985 = 3
            w1002 = 7
            w1004 = 6
            w1018 = 1
            w1012 = 2
            w1010 = 3
            w1008 = 4
            w1006 = 5
            w1014 = 0
            # "1100 - 1150,  1750-1800,  2250-2600, 3975--4025,  4400--4500,  6175--6275"
            n584 = event-data() -> ()  [unwired: 7 out]
            n585 = case shown="0, Default" "Substrate" {
              tunnel: [dbl[] [328.16, 495.4, 753.66, 1157.4, 1313.3, 2003.9, 2014.8, 2175.7, 2822.6, 3043.4, 3398.1, 3767.8, 4232.0, 4806.5, 4837.8, 4986.6, 5573.5, 6031.7, 6389.6, 6767.0, 7063.3, 7348.2, 8139.4, 8697.8, 8729.1, 8786.8, 8920.1, 10050.0, 10347.0] dbl[] [1092.3, 1649.9, 2505.8, 3847.7, 4361.2, 6645.1, 6683.3, 7225.3, 9346.1, 10072.0, 11259.0, 12454.0, 13972.0, 15881.0, 15961.0, 16483.0, 18354.0, 19859.0, 21048.0, 22299.0, 23198.0, 24139.0, 26725.0, 28486.0, 28665.0, 28795.0, 29295.0, 32885.0, 33819.0] dbl[] [2760.1, 4168.9, 6298.4, 9640.0, 10894.0, 16481.0, 16575.0, 17940.0, 22992.0, 24705.0, 27613.0, 30365.0, 33870.0, 37411.0, 38418.0, 38537.0, 39856.0, 41993.0, 43948.0, 47449.0, 48423.0, 50180.0, 53083.0, 54835.0, 57044.0, 57205.0, 62763.0, 64874.0, 66442.0]] -> w982
              tunnel: [0.1 0.5 2.0] -> w1024
              tunnel: [11.0 35.0 70.0] -> w1023
              tunnel: [u8[] [1, 3, 5, 6, 9, 12, 15, 18, 22, 26, 29] u8[] [1, 3, 5, 6, 9, 12, 15, 18, 22, 26, 29] u8[] [1, 3, 5, 6, 9, 12, 16, 20, 25, 0, 0]] -> w994
              tunnel: [u8[] [1, 3, 4, 5, 6, 7, 9, 10, 11, 12, 13, 14, 15, 17, 18, 19, 20, 21, 22, 23, 24, 25, 26, 28, 29] u8[] [1, 3, 4, 5, 6, 7, 9, 10, 11, 12, 13, 14, 15, 17, 18, 19, 20, 21, 22, 23, 24, 25, 26, 28, 29] u8[] [1, 3, 4, 5, 6, 7, 9, 10, 11, 12, 13, 14, 15, 16, 19, 20, 21, 22, 23, 24, 25, 26, 27, 28, 29]] -> w983
              frame 0, Default {
              }
              frame 1 {
              }
              frame 2 {
              }
            }
            "All Modes" <- w982
            n586 = property on="fMaxPlot" class="DigNum (strict)"("Val(Sgnl)"=w1023) -> ()  [unwired: 2 in, 2 out]
            n587 = property on="fMinPlot" class="DigNum (strict)"("Val(Sgnl)"=w1024) -> ()  [unwired: 2 in, 2 out]
            n588 = for {
              tunnel: w983 -> [w1050] mode=indexing
              tunnel: w982 -> [w1051]
              tunnel: [w1049] -> w984 mode=indexing
              n589 = Index Array(array=w1051, index=w1050) -> (element=w1049:dbl)
            }
            "Nodal Modes" <- w984
            n590 = for {
              tunnel: w994 -> [w1053] mode=indexing
              tunnel: w982 -> [w1054]
              tunnel: [w1052] -> w986 mode=indexing
              n591 = Index Array(array=w1054, index=w1053) -> (element=w1052:dbl)
            }
            "Shear Modes" <- w986
            n592 = for {
              N: 2 -> [_]
              tunnel: w994 -> [w1059]
              tunnel: [w1055] -> w989 mode=indexing
              tunnel: [w1056] -> w993 mode=indexing
              tunnel: w982 -> [w1058]
              i -> [w1057]
              n593 = for {
                N: 8 -> [_]
                tunnel: [w1067] -> w1056 mode=indexing
                tunnel: w1057 -> [w1066]
                tunnel: w1059 -> [w1065] mode=indexing
                tunnel: w1058 -> [w1062]
                tunnel: [w1061] -> w1055 mode=indexing
                i -> [w1064]
                n594 = case shown="0, Default" w1066 {
                  tunnel: [w1076 w1078] -> w1063
                  tunnel: w1065 -> [_ w1078]
                  tunnel: w1064 -> [w1074 _]
                  tunnel: w1062 -> [w1075 w1080]
                  tunnel: [w1073 w1077] -> w1061
                  frame 0, Default {
                    n595 = Increment(x=w1074) -> (x+1=w1076:i32)
                    n596 = Index Array(array=w1075, index=w1074) -> (element=w1073:dbl)
                  }
                  frame 1 {
                    n597 = Decrement(x=w1078) -> (x-1=w1079:u8)
                    n598 = Index Array(array=w1080, index=w1079) -> (element=w1077:dbl)
                  }
                }
                n599 = Number To Decimal String(number=w1063) -> (decimal integer string=w1071:string)  [unwired: 1 in]
                n600 = Number To Decimal String(number=w1061) -> (decimal integer string=w1069:string)  [unwired: 1 in]
                n601 = Concatenate Strings("Mode ", w1071, ": ", w1069, " Hz (FEM)") -> (w1067:string)
              }
            }
            "PlotLabelArray" <- w993
            "PlotFreqArray" <- w989
            n602 = Array Subset(array=w982, index=0, length=w985) -> (→"Modes 1-3":dbl[])
            n603 = Array Subset(array=w982, index=3, length=w985) -> (→"Modes 4-6":dbl[])
            n604 = Array Subset(array=w982, index=6, length=w985) -> (→"Modes 7-9":dbl[])
            n605 = Array Subset(array=w982, index=9, length=w985) -> (→"Modes 10-12":dbl[])
            n606 = Array Size(array=w993) -> (size(s)=→"PlotLabelSize":i32[])
            n607 = Array Size(array=w989) -> (size(s)=→"PlotModeSize":i32[])
            n608 = Index Array(array=w989, index (row)="Sample Modes") -> (element=w987:dbl[])  [unwired: 1 in]
            n609 = Index Array(array=w993, index (row)="Sample Modes") -> (element=w990:string[])  [unwired: 1 in]
            n610 = Divide(x="Range (%)", y=100.0) -> (x/y=w1045:dbl)
            n611 = Multiply(x="Mode Scale", y=w987) -> (x*y=w1016:dbl[])
            n612 = Increment(x=w1045) -> (x+1=w1015:dbl)
            n613 = Subtract(x=1.0, y=w1045) -> (x-y=w1044:dbl)
            n614 = Multiply(x=w1016, y=w1044) -> (x*y=w1043:dbl[])
            n615 = Multiply(x=w1016, y=w1015) -> (x*y=w1034:dbl[])
            n616 = Index Array(array=w990, index=w1014) -> (element=→"Plot1Label":string)
            n617 = Index Array(array=w1034, index=w1014) -> (element=w1033:dbl)
            n618 = Index Array(array=w1043, index=w1014) -> (element=w1042:dbl)
            n619 = property on="Plot1" class="WFGraph (strict)"("XScale.Maximum"=w1033) -> ()  [unwired: 2 in, 2 out]
            n620 = property on="Plot1" class="WFGraph (strict)"("XScale.Minimum"=w1042) -> ()  [unwired: 2 in, 2 out]
            n621 = Index Array(array=w990, index=w1018) -> (element=→"Plot2Label":string)
            n622 = Index Array(array=w1043, index=w1018) -> (element=w1041:dbl)
            n623 = Index Array(array=w1034, index=w1018) -> (element=w1032:dbl)
            n624 = property on="Plot2" class="WFGraph (strict)"("XScale.Minimum"=w1041) -> ()  [unwired: 2 in, 2 out]
            n625 = property on="Plot2" class="WFGraph (strict)"("XScale.Maximum"=w1032) -> ()  [unwired: 2 in, 2 out]
            n626 = Index Array(array=w990, index=w1012) -> (element=→"Plot3Label":string)
            n627 = Index Array(array=w1043, index=w1012) -> (element=w1040:dbl)
            n628 = Index Array(array=w1034, index=w1012) -> (element=w1031:dbl)
            n629 = property on="Plot3" class="WFGraph (strict)"("XScale.Minimum"=w1040) -> ()  [unwired: 2 in, 2 out]
            n630 = property on="Plot3" class="WFGraph (strict)"("XScale.Maximum"=w1031) -> ()  [unwired: 2 in, 2 out]
            n631 = Index Array(array=w990, index=w1010) -> (element=→"Plot4Label":string)
            n632 = Index Array(array=w1034, index=w1010) -> (element=w1030:dbl)
            n633 = Index Array(array=w1043, index=w1010) -> (element=w1039:dbl)
            n634 = property on="Plot4" class="WFGraph (strict)"("XScale.Maximum"=w1030) -> ()  [unwired: 2 in, 2 out]
            n635 = property on="Plot4" class="WFGraph (strict)"("XScale.Minimum"=w1039) -> ()  [unwired: 2 in, 2 out]
            n636 = Index Array(array=w990, index=w1008) -> (element=→"Plot5Label":string)
            n637 = Index Array(array=w1043, index=w1008) -> (element=w1038:dbl)
            n638 = Index Array(array=w1034, index=w1008) -> (element=w1029:dbl)
            n639 = property on="Plot5" class="WFGraph (strict)"("XScale.Minimum"=w1038) -> ()  [unwired: 2 in, 2 out]
            n640 = property on="Plot5" class="WFGraph (strict)"("XScale.Maximum"=w1029) -> ()  [unwired: 2 in, 2 out]
            n641 = Index Array(array=w990, index=w1006) -> (element=→"Plot6Label":string)
            n642 = Index Array(array=w1034, index=w1006) -> (element=w1028:dbl)
            n643 = Index Array(array=w1043, index=w1006) -> (element=w1037:dbl)
            n644 = property on="Plot6" class="WFGraph (strict)"("XScale.Minimum"=w1037) -> ()  [unwired: 2 in, 2 out]
            n645 = property on="Plot6" class="WFGraph (strict)"("XScale.Maximum"=w1028) -> ()  [unwired: 2 in, 2 out]
            n646 = Index Array(array=w990, index=w1004) -> (element=→"Plot7Label":string)
            n647 = Index Array(array=w1043, index=w1004) -> (element=w1036:dbl)
            n648 = Index Array(array=w1034, index=w1004) -> (element=w1027:dbl)
            n649 = property on="Plot7" class="WFGraph (strict)"("XScale.Minimum"=w1036) -> ()  [unwired: 2 in, 2 out]
            n650 = property on="Plot7" class="WFGraph (strict)"("XScale.Maximum"=w1027) -> ()  [unwired: 2 in, 2 out]
            n651 = Index Array(array=w990, index=w1002) -> (element=→"Plot8Label":string)
            n652 = Index Array(array=w1043, index=w1002) -> (element=w1035:dbl)
            n653 = Index Array(array=w1034, index=w1002) -> (element=w1026:dbl)
            n654 = property on="Plot8" class="WFGraph (strict)"("XScale.Minimum"=w1035) -> ()  [unwired: 2 in, 2 out]
            n655 = property on="Plot8" class="WFGraph (strict)"("XScale.Maximum"=w1026) -> ()  [unwired: 2 in, 2 out]
          }
          event "QUIT": Mouse Down {
            n656 = event-data() -> ()  [unwired: 4 out]
            n657 = call <vilib>:"Three Button Dialog.vi"("Window Title (\"\")"="Quit or Stop?", "Right Button Text (\"Cancel\")"="Cancel", "Center Button Text (\"No\")"="Stop", "Left Button Text (\"Yes\")"="Quit", "message"="Stop operation (debug) or Quit the applcation?") -> ("Which Button?"=w1098:T9)  [unwired: 6 out]
            n658 = case shown="\"Center Button\"" w1098 {
              tunnel: [TRUE TRUE FALSE FALSE] -> w1096
              frame "Left Button", Default {
              }
              frame "Center Button" {
              }
              frame "Right Button" {
              }
              frame "Window Close" {
              }
            }
            n659 = Greater Than 0?(x=w1098) -> (x > 0?=w1097:bool)
          }
          event "Unit", "Type": Value Change {
            n660 = event-data() -> ()  [unwired: 7 out]
            n661 = Equal To 0?(x="Type") -> (x = 0?=w1109:bool)
            n662 = Equal To 0?(x="Unit") -> (x = 0?=w1111:bool)
            n663 = case shown="False" w1111 {
              tunnel: [w1114 w1117] -> w1108
              tunnel: w1109 -> [w1113 w1118]
              frame False {
                n664 = case shown="False" w1113 {
                  tunnel: ["Power Density [Rad / rHz]" "Power [Rad]"] -> w1114
                  frame False {
                  }
                  frame True {
                  }
                }
              }
              frame True {
                n665 = case shown="True" w1118 {
                  tunnel: ["Power Density [V / V_total / rHz]" "Power [V / V_total]"] -> w1117
                  frame False {
                  }
                  frame True {
                  }
                }
              }
            }
            n666 = property on="Plot5" class="WFGraph (strict)"("YScale.NameLbl.Text"=w1108) -> ()  [unwired: 2 in, 2 out]
            n667 = property on="Plot6" class="WFGraph (strict)"("YScale.NameLbl.Text"=w1108) -> ()  [unwired: 2 in, 2 out]
            n668 = property on="Plot8" class="WFGraph (strict)"("YScale.NameLbl.Text"=w1108) -> ()  [unwired: 2 in, 2 out]
            n669 = property on="Plot7" class="WFGraph (strict)"("YScale.NameLbl.Text"=w1108) -> ()  [unwired: 2 in, 2 out]
            n670 = property on="Plot3" class="WFGraph (strict)"("YScale.NameLbl.Text"=w1108) -> ()  [unwired: 2 in, 2 out]
            n671 = property on="Plot4" class="WFGraph (strict)"("YScale.NameLbl.Text"=w1108) -> ()  [unwired: 2 in, 2 out]
            n672 = property on="Plot2" class="WFGraph (strict)"("YScale.NameLbl.Text"=w1108) -> ()  [unwired: 2 in, 2 out]
            n673 = property on="Plot1" class="WFGraph (strict)"("YScale.NameLbl.Text"=w1108) -> ()  [unwired: 2 in, 2 out]
            n674 = property on="PSD Y" class="WFGraph (strict)"("YScale.NameLbl.Text"=w1108) -> ()  [unwired: 2 in, 2 out]
            n675 = property on="PSD X" class="WFGraph (strict)"("YScale.NameLbl.Text"=w1108) -> ()  [unwired: 2 in, 2 out]
          }
        }
      }
    }
    frame #2 {
      n676 = case shown="False" w1121 {
        frame False {
          n677 = Quit LabVIEW() -> ()  [unwired: 1 out]
        }
        frame True {
          n678 = Stop() -> ()  [unwired: 1 out]
        }
      }
    }
  }
